vi "Cascade front panel.vi"() -> ()   [LabVIEW 2016]
uses:
  SDI-12/Sonde Vertical Graph.ctl
  Waterloo DAQ/controls/Vertical Chart.ctl
  activeXtest/activeXtest 2015 Folder/sample data row cluster.ctl
  activeXtest/activeXtest 2015 Folder/sonde cluster.ctl
  Groundwater header.ctl
  Waterloo DAQ/controls/MCC DAQ Setup.ctl
  Waterloo DAQ/controls/Aux Sensor.ctl
  KPRO_2016 subvis/Control 2.ctl
  KPRO_2016 subvis/Control 9.ctl
  KPRO_2016 subvis/Graph Controls 2.ctl
  KPRO_2016 subvis/Ik control.ctl
  KPRO_2016 subvis/Ion Slope Control 8.ctl
  KPRO_2016 subvis/Depth Control.ctl
  KPRO_2016 subvis/SS Control 7.ctl
  Waterloo DAQ/controls/Action Control 1.ctl
  <extravilib>/ChannelInstances/One Element Stream-t'Action Control 1.ctl'/Instantiate.vi
  <extravilib>/ChannelInstances/One Element Stream-t'Action Control 1.ctl'/Endpoint.vi
  <vilib>/ULx/Create Channel.llb/ULx Create Channel (AI-Voltage-Basic).vi
  <vilib>/ULx/Read.llb/ULx Read (Analog DBL 1Chan 1Samp).vi
  C:/Program Files (x86)/National Instruments/LabVIEW 2016/vi.lib/ULx/ULx_LV.dll
  <vilib>/Utility/NIReport.llb/NI_report.lvclass
  <vilib>/Utility/config.llb/NI_LVConfig.lvlib
  <extravilib>/ChannelInstances/One Element Stream-t'Action Control 1.ctl'.lvlib
panel:
  out "Feet of Stainless 2":i32
  out "Feet of\nStainless to be\nUsed (Count)":i32
  in  "SS In":i32
  in  "Record Continuous Samples":bool
  out "Current Time (s)":dbl
  in  "Sample Sheet Data Row Cluster 2":T1={"Head"=0.0, "Depth"=0.0, "comment string"="", "Sonde Data Cluster"={"Cumulative\nVolume"=100.0, "Specific\nConductance"=2.0, "Dissolved\nOxygen"=3.0, "pH"=4.0, "ORP"=5.0, "Temp"=26.0, "Salinity"=7.0}} {"Sonde Data Cluster"."Salinity" format="%_3g"; "Sonde Data Cluster"."Temp" format="%_2g"; "Sonde Data Cluster"."ORP" format="%_4g"; "Sonde Data Cluster"."pH" format="%_4g"; "Sonde Data Cluster"."Dissolved\nOxygen" format="%_4g"; "Sonde Data Cluster"."Specific\nConductance" format="%_4g"; "Sonde Data Cluster"."Cumulative\nVolume" format="%#_4g"}
  in  "stop":bool
  in  "Write Data to Spreadsheet":bool
  in  "Sample Not Collected":bool
  in  "Record Single Sample":bool
  in  "Tab Control":T3(tab)
  out "12V Voltage Monitor":dbl format="%_3f"
  out "Found Quanta Sonde Com Port":refnum<visa-resource-name>
  in  "Temporary Data Files Directory":path=path "D:/Cascade/Data/Raw Sonde Data"
  in  "Data File Directory":path=path "D:/Cascade/Data/Excel Reports"
  out "Quanta Sonde found?":bool
  in  "report file path":path=path "D:/Cascade/templates/Groundwater Profiling Log_empty_2.xlsx"
  in  "template file path":path=path "D:/Cascade/templates/Groundwater Profiling Log_empty_labview_template.xlsx"
  in  "Config File Path":path=path "D:/Cascade/Data/config files/DAQ Setup Config.ini"
  in  "Read Configuration File?":bool=TRUE
  out "H-4191 Adapter found":bool
  in  "Save Configuration File?":bool
  out "Sonde Communication Error Out":errorcluster
  in  "Search for Comm Ports?":bool=TRUE
  in  "USB Serial Port Manual Entry":refnum<visa-resource-name>="COM13"
  in  "MCC USB-DAQ Setup":T4={"Device Name in InstaCal"="Dev0", "Omega Pressure Sensor"={"DAQ Channel"=2.0, "Output Voltage Range"=1, "Enabled"=TRUE, "Description"="Uphole Pressure"}, "McMillian 102 Flowmeter"={"DAQ Channel"=11.0, "Output Voltage Range"=1, "Enabled"=TRUE, "Description"="Flow"}, "DHT Pressure Sensor"={"DAQ Channel"=3.0, "Output Voltage Range"=1, "Enabled"=TRUE, "Description"="Downhole Pressure"}, "Top String Pot"={"DAQ Channel"=0.0, "Output Voltage Range"=0, "Enabled"=TRUE, "Description"="Top String Pot"}, "String Pot Signal"={"DAQ Channel"=1.0, "Output Voltage Range"=0, "Enabled"=TRUE, "Description"="String Pot"}, "Aux Sensor 1"={"DAQ Channel"=5.0, "Output Voltage Range"=1, "Enabled"=FALSE, "Description"="Aux 1"}, "Aux Sensor 2"={"DAQ Channel"=6.0, "Output Voltage Range"=1, "Enabled"=FALSE, "Description"="Aux 2"}, "Aux Sensor 3"={"DAQ Channel"=7.0, "Output Voltage Range"=1, "Enabled"=TRUE, "Description"="Aux 3"}, "Voltage Monitor"={"DAQ Channel"=8.0, "Output Voltage Range"=0, "Enabled"=TRUE, "Description"="9V Monitor"}} {"Voltage Monitor"."Output Voltage Range" items=["+/-10 V Range", "+/-5 V Range", "+/-2.5V Range", "+/-1.25 V Range", "+/-0.625 V Range", "+/-0.3125 V Range", "+/-0.1562V Range", "+/-0.078125 V Range"]; "Aux Sensor 3"."Output Voltage Range" items=["+/-10 V Range", "+/-5 V Range", "+/-2.5V Range", "+/-1.25 V Range", "+/-0.625 V Range", "+/-0.3125 V Range", "+/-0.1562V Range", "+/-0.078125 V Range"]; "Aux Sensor 2"."Output Voltage Range" items=["+/-10 V Range", "+/-5 V Range", "+/-2.5V Range", "+/-1.25 V Range", "+/-0.625 V Range", "+/-0.3125 V Range", "+/-0.1562V Range", "+/-0.078125 V Range"]; "Aux Sensor 1"."Output Voltage Range" items=["+/-10 V Range", "+/-5 V Range", "+/-2.5V Range", "+/-1.25 V Range", "+/-0.625 V Range", "+/-0.3125 V Range", "+/-0.1562V Range", "+/-0.078125 V Range"]; "String Pot Signal"."Output Voltage Range" items=["+/-10 V Range", "+/-5 V Range", "+/-2.5V Range", "+/-1.25 V Range", "+/-0.625 V Range", "+/-0.3125 V Range", "+/-0.1562V Range", "+/-0.078125 V Range"]; "Top String Pot"."Output Voltage Range" items=["+/-10 V Range", "+/-5 V Range", "+/-2.5V Range", "+/-1.25 V Range", "+/-0.625 V Range", "+/-0.3125 V Range", "+/-0.1562V Range", "+/-0.078125 V Range"]; "DHT Pressure Sensor"."Output Voltage Range" items=["+/-10 V Range", "+/-5 V Range", "+/-2.5V Range", "+/-1.25 V Range", "+/-0.625 V Range", "+/-0.3125 V Range", "+/-0.1562V Range", "+/-0.078125 V Range"]; "McMillian 102 Flowmeter"."Output Voltage Range" items=["+/-10 V Range", "+/-5 V Range", "+/-2.5V Range", "+/-1.25 V Range", "+/-0.625 V Range", "+/-0.3125 V Range", "+/-0.1562V Range", "+/-0.078125 V Range"]; "Omega Pressure Sensor"."Output Voltage Range" items=["+/-10 V Range", "+/-5 V Range", "+/-2.5V Range", "+/-1.25 V Range", "+/-0.625 V Range", "+/-0.3125 V Range", "+/-0.1562V Range", "+/-0.078125 V Range"]}
  out "Rate":dbl=1000.0 caption="Sample Rate (Hz)"
  out "Number of Channels":u16
  in  "Channel Data Rate S/s":dbl=3720.0 format="%#_13g"
  out "Descriptions":string[](array[string])
  out "Raw Voltages":dbl[](array[numeric])
  out "9V Voltage Monitor":dbl
  in  "Record DAQ Raw Voltages":bool
  in  "Groundwater Header":T6
  out "Worksheet Names":string[](array[string])
  in  "Current Sheet":i32=1
  out "row max value":i32
  out "last occupied cell's name":string
  out "Current Sample Sheet":string="Sample 1"
  in  "Cluster":T7={"Profile ID"="WP-01", "Hole Id"="HOLE_001"}
  out "Sonde Data Array":string[][](array[string])
  out "Table Label":string="Data from Sample Sheet %d from Excel File"
  out "Sonde Data Display":T8
  out "Temperature":cluster{"Y":dbl[], "Y":dbl[]}[](graph)
  in  "Record Reason":bool
  in  "Select Reasons to Record Data":u16(ring) items=["Per Client Request", "Timed Out", "Sample stopped flowing", "Equipment Issue"]
  out "SC  Reference\nCalibrate Response":bool
  out "DO  Reference\nCalibrate Response":bool
  in  "Salinity \nReference":dbl
  out "Salinity  Reference\nCalibrate Response":bool
  out "ORP  Reference\nCalibrate Response":bool
  in  "SC \nReference":dbl
  in  "DO \nReference":dbl
  in  "ORP Reference":dbl
  in  "pH Reference":dbl
  in  "pH Zero":dbl
  in  "Record  SC Calibration":bool
  in  "Record DO Calibration":bool
  in  "Record Salinity Calibration":bool
  in  "Record ORP Calibration":bool
  in  "Record pH Calibration Reference":bool
  in  "Record pH Calibration Zero":bool
  out "pH Zero \nCalibrate Response":bool
  out "pH  Reference\nCalibrate Response":bool
  in  "Ion Offset":dbl format="%.2f"
  in  "Ion Slope":dbl=44.04 format="%.2f"
  in  "Pressure \nSlope":dbl=24.27199935913086 format="%.2f"
  in  "Flow Slope":dbl=37.99800109863281 format="%.2f"
  in  "String Pot \nSlope":dbl=1.7339999675750732 format="%.2f"
  out "Slug Test\nIndicator copy":bool
  out "KPRO Test\nIndicator":bool
  in  "Start\nST":bool
  in  "Finish Tests":bool
  in  "Start  KPRO":bool
  in  "Feet of Stainless":i32=40
  out "Cluster 7":T10={"Flow"=0.21081600494384767, "Zeroed \nPressure"=74.74207969932556, "Ik"=0.003788962123473114, "Current Depth"=-100.6, "Feet of Stainless"=40, "Start Depth"=0.0, "Hole_Name_Path"=path "C:/e"} {"Start Depth" format="%.2f"; "Current Depth" format="%.2f"; "Ik" format="%.2f"; "Zeroed \nPressure" format="%.2f"; "Flow" format="%.2f"}
  in  "Cluster 2":T11={"Ion Slope"=44.04, "Ion Offset"=0.0, "Height of Sample Box"=0.0, "Last_Pressure_Slope"=48.27000045776367, "Last_Flow_Slope"=39.040000915527344, "Last_String_Pot_Slope"=1.6619999408721924} {"Last_String_Pot_Slope" format="%.2f"; "Last_Flow_Slope" format="%.2f"; "Last_Pressure_Slope" format="%.2f"; "Height of Sample Box" format="%.2f"; "Ion Offset" format="%.2f"; "Ion Slope" format="%.2f"}
  in  "Slope Cluster":T12={"Total Volume"=0.0, "String Pot Slope"=1.6619999408721924, "Flow Slope"=39.040000915527344, "Pressure Slope"=48.27000045776367, "Depth to Water Table"=-0.0, "Atmospheric Pressure"=32.22022530555725, "Reservoir Pressure"=-0.004827000045779073} {"Reservoir Pressure" format="%.2f"; "Atmospheric Pressure" format="%.2f"; "Depth to Water Table" format="%.2f"; "Pressure Slope" format="%.2f"; "Flow Slope" format="%.2f"; "String Pot Slope" format="%.2f"; "Total Volume" format="%.2f"}
  in  "Cluster 6":T13
  out "Cluster 4":T14={"Real Time - Depth vs. lk "={[0.003788962123473114, 0.0037174584307500765, 0.0037174584307500765, 0.0037174584307500765, 0.0037174584307500765, 0.003788962123473114], [-100.1, -100.2, -100.3, -100.4, -100.5, -100.6]}, "Real Time - Depth vs. lk  2"={[0.003788962123473114, 0.0037174584307500765, 0.0037174584307500765, 0.0037174584307500765, 0.0037174584307500765, 0.003788962123473114], [-100.1, -100.2, -100.3, -100.4, -100.5, -100.6]}, "Real Time - Depth vs. lk  2"={[0.003788962123473114, 0.0037174584307500765, 0.0037174584307500765, 0.0037174584307500765, 0.0037174584307500765, 0.003788962123473114], [-100.1, -100.2, -100.3, -100.4, -100.5, -100.6]}, "Ik "=0.003788962123473114, "Current Depth"=-100.6} {"Current Depth" format="%.2f"; "Ik" format="%.2f"}
  in  "Cluster 3":T15={"Cumulative - Depth vs. Ik"={[], []}, "Real Time - Depth vs. lk "={[0.003788962123473114, 0.0037174584307500765, 0.0037174584307500765, 0.0037174584307500765, 0.0037174584307500765, 0.003788962123473114], [-100.1, -100.2, -100.3, -100.4, -100.5, -100.6]}, "Cumulative - Depth vs. Drive"={[], []}, "Real Time - Depth vs. Drive"={[0.02036245163917736, 0.125, 0.16666666666666674, 0.16666666666666663, 0.16666666666666663, 0.16666666666666663], [-100.1, -100.2, -100.3, -100.4, -100.5, -100.6]}}
  out "DAQ Error":errorcluster
  out "Initialization Finished":bool=TRUE
  out "Stop":bool
  out "error out":errorcluster
  in  "error in (no error)":errorcluster
  out "producer loop":i32
  out "consumer loop":i32
  out "Active Channel Array":string[](array[string])
  out "delimited string":string
  out "Voltage Range":dbl[](array[numeric])
  out "Stop 2":bool
  # "Instructions for Sonde Calibration:\n1.  Use the Record Single Point to Record the Data prior to start of\ncalibration procedure to record the initial points to the excel worksheet.\n2.  pH Calibration is a 2 step process:  A pH standard between 6.8 and 7.2 is treated as the “zero”\nand all other values are treated as the “slope”. First calibrate “zero”, then  add a second to calibrate “slope”. \n3.  Specific Conductance:  Wait for the specific conductance readings to stabilize in the calibration solution, which may\nrequire one or two minutes."
  # "String Pot"
  # "Use Incr"
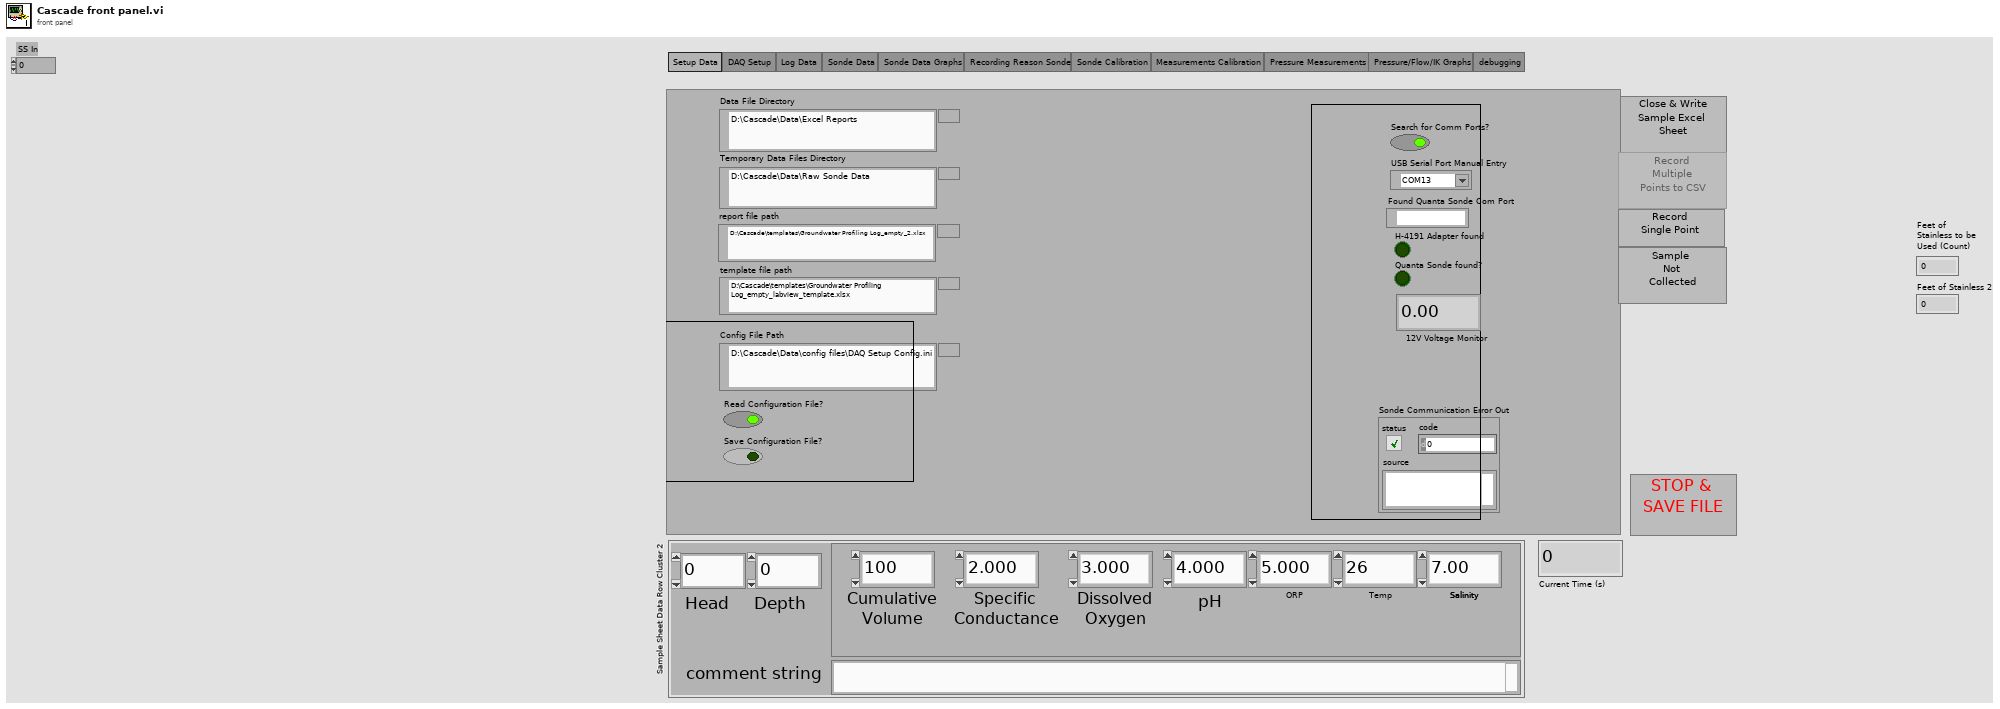
[diagram p1: front panel]
types:
  T1 = typedef "sample data row cluster.ctl" = cluster{"Head":dbl, "Depth":dbl, "comment string":string, "Sonde Data Cluster":T2}
  T2 = typedef "sonde cluster.ctl" = cluster{"Cumulative\nVolume":dbl, "Specific\nConductance":dbl, "Dissolved\nOxygen":dbl, "pH":dbl, "ORP":dbl, "Temp":dbl, "Salinity":dbl}
  T3 = enum32{"Setup Data", "DAQ Setup", "Log Data", "Sonde Data", "Sonde Data Graphs", "Recording Reason Sonde", "Sonde Calibration", "Measurements Calibration", "Pressure Measurements", "Pressure/Flow/IK Graphs", "debugging"}
  T4 = typedef "MCC DAQ Setup.ctl" = cluster{"Device Name in InstaCal":string, "Omega Pressure Sensor":T5, "McMillian 102 Flowmeter":T5, "DHT Pressure Sensor":T5, "Top String Pot":T5, "String Pot Signal":T5, "Aux Sensor 1":T5, "Aux Sensor 2":T5, "Aux Sensor 3":T5, "Voltage Monitor":T5}
  T5 = typedef "Aux Sensor.ctl" = cluster{"DAQ Channel":dbl, "Output Voltage Range":u16, "Enabled":bool, "Description":string}
  T6 = typedef "Groundwater header.ctl" = cluster{"Location":string, "Date Finished":string, "CTS":string, "sampler":string, "Kpro box Serial ":string, "Sonde Serial":string, "Drilling Contractor":string, "Ave Depth to Water":string, "Gas/Peri Pump":string, "Atmospheric Pressure":string, "KPRO N2 Pressure":string, "Gas Drive N2 Pressure":string}
  T7 = typedef "Control 9.ctl" = cluster{"Profile ID":string, "Hole Id":string}
  T8 = typedef "Sonde Vertical Graph.ctl" = cluster{"pH":T9, "Conductance":T9, "Salinity":T9, "DO % Saturation":T9, "DO mg/L":T9, "ORP":T9}
  T9 = typedef "Vertical Chart.ctl" = cluster{"Y":dbl[], "Y":dbl[]}[]
  T10 = typedef "SS Control 7.ctl" = cluster{"Flow":dbl, "Zeroed \nPressure":dbl, "Ik":dbl, "Current Depth":sgl, "Feet of Stainless":i32, "Start Depth":sgl, "Hole_Name_Path":path}
  T11 = typedef "Ion Slope Control 8.ctl" = cluster{"Ion Slope":dbl, "Ion Offset":dbl, "Height of Sample Box":dbl, "Last_Pressure_Slope":dbl, "Last_Flow_Slope":dbl, "Last_String_Pot_Slope":dbl}
  T12 = typedef "Control 2.ctl" = cluster{"Total Volume":dbl, "String Pot Slope":dbl, "Flow Slope":dbl, "Pressure Slope":dbl, "Depth to Water Table":dbl, "Atmospheric Pressure":dbl, "Reservoir Pressure":dbl}
  T13 = typedef "Depth Control.ctl" = cluster{"Depth mode":bool, "Increment\nButton":bool}
  T14 = typedef "Ik control.ctl" = cluster{"Real Time - Depth vs. lk ":cluster{dbl[], dbl[]}, "Real Time - Depth vs. lk  2":cluster{dbl[], dbl[]}, "Real Time - Depth vs. lk  2":cluster{dbl[], dbl[]}, "Ik ":dbl, "Current Depth":sgl}
  T15 = typedef "Graph Controls 2.ctl" = cluster{"Cumulative - Depth vs. Ik":cluster{dbl[], dbl[]}, "Real Time - Depth vs. lk ":cluster{dbl[], dbl[]}, "Cumulative - Depth vs. Drive":cluster{dbl[], dbl[]}, "Real Time - Depth vs. Drive":cluster{dbl[], dbl[]}}
  T16 = typedef "Action Control 1.ctl" = enum16{"TimeOut", "Continuous  Data", "Init", "Exit", "Acq. Single Point", "Write Sample Sheet", "Acq. DAQ data", "Sample Not Collected", "Record Reason", "pH Calibration Zero", "pH Calibration Standard", "ORP Calibration Standard", "Salinity Calibration Standard", "DO Calibration Standard", "SC Calibration Standard"}
  T17 = typedef "NI_LVConfig.lvlib/Config Data RefNum.ctl" = refnum<k1>
  T18 = enum8{"Enabled", "Disabled", "Disabled and Grayed Out"}
  T19 = typedef "One Element Stream-t'Action Control 1.ctl'.lvlib/)Channel.ctl" = refnum<queue>
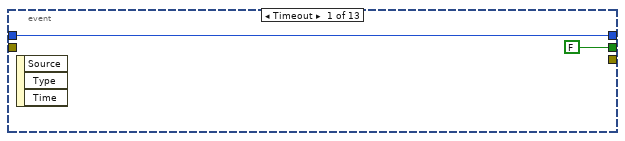
[diagram p2: hidden frame]
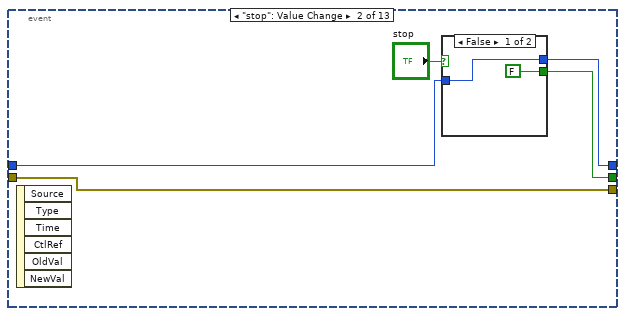
[diagram p3: hidden frame]
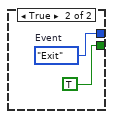
[diagram p4: hidden frame]
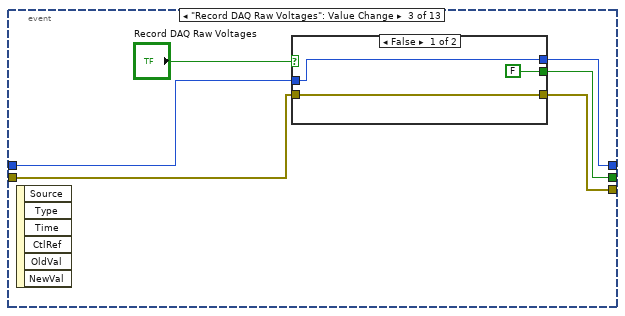
[diagram p5: hidden frame]
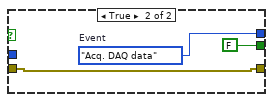
[diagram p6: hidden frame]
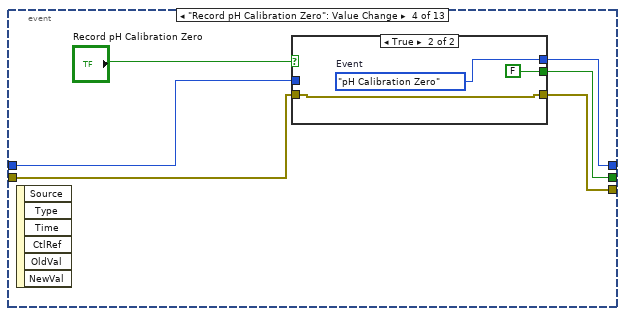
[diagram p7: hidden frame]
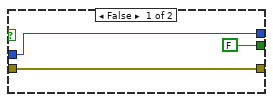
[diagram p8: hidden frame]
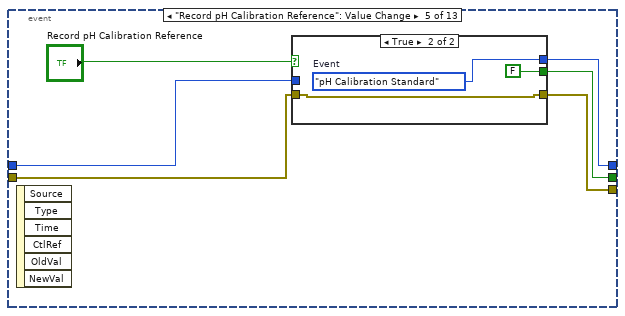
[diagram p9: hidden frame]
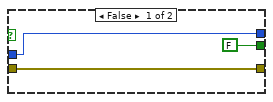
[diagram p10: hidden frame]
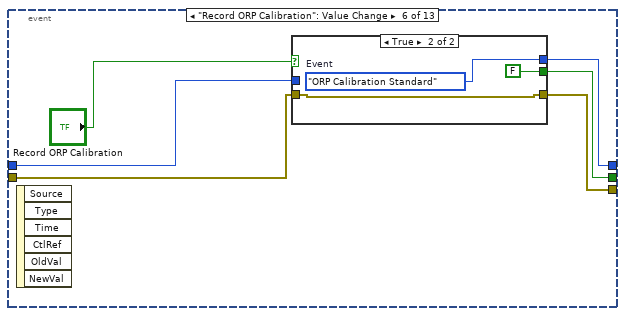
[diagram p11: hidden frame]
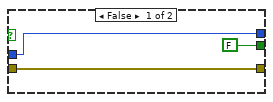
[diagram p12: hidden frame]
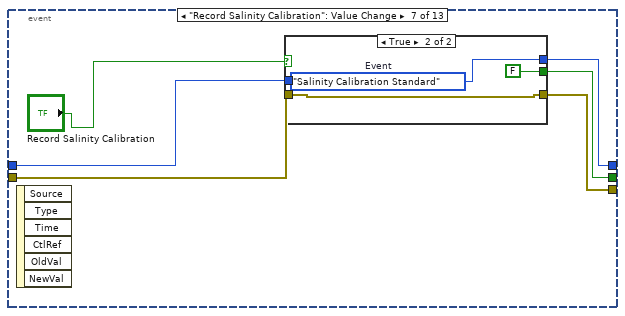
[diagram p13: hidden frame]
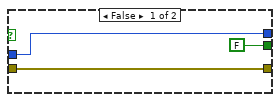
[diagram p14: hidden frame]
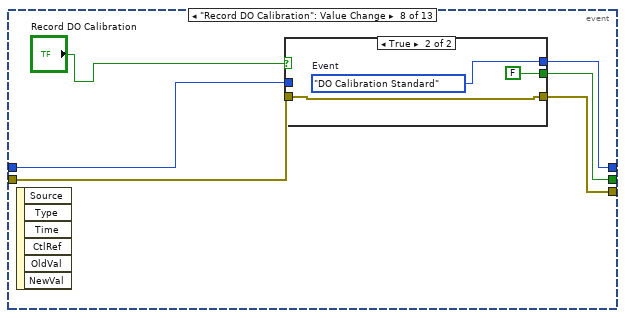
[diagram p15: hidden frame]
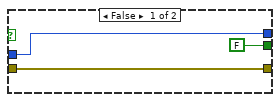
[diagram p16: hidden frame]
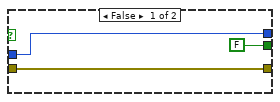
[diagram p17: hidden frame]
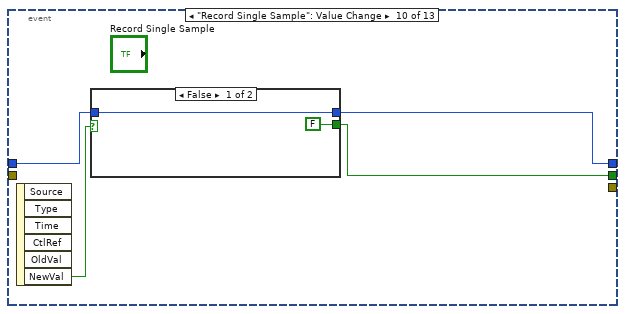
[diagram p18: hidden frame]
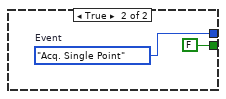
[diagram p19: hidden frame]
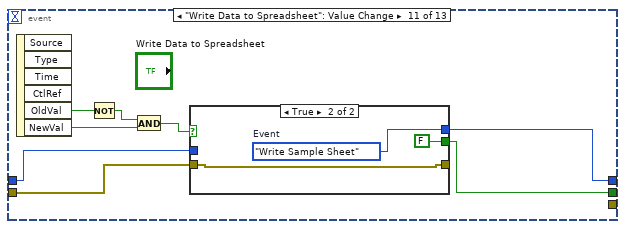
[diagram p20: hidden frame]
diagram:
  w7 = Action_Control_1."Init"  # Event
  # "For calibrate command (XC) on SDI-12 address ‘a’, P is pH, C is specific conductance, S is\nsalinity or TDS, % is DO %Saturation, O is DO mg/L, R is ORP, D is depth, B is\nbarometric pressure, and t is TDS scale factor."
  n1 = flat-sequence {
    tunnel: [w31] -> w10
    tunnel: [w63] -> w16
    tunnel: w10 -> [w63]
    tunnel: [w59] -> w6
    tunnel: [w74] -> w26
    tunnel: w16 -> [w71]
    tunnel: [w71] -> w11
    tunnel: w26 -> [w130]
    tunnel: [w102] -> w24
    tunnel: [w106] -> w22
    tunnel: [w113] -> w17
    tunnel: [w112] -> w19
    tunnel: [w111] -> w20
    tunnel: [w104] -> _
    tunnel: [w100] -> w25
    tunnel: ["Feet of Stainless"] -> w5
    tunnel: [w97] -> w4
    tunnel: [w96] -> w3
    frame #0 {
      n2 = flat-sequence {
        tunnel: [w35] -> w31
        tunnel: "error in (no error)" -> [w34]
        frame #0 {
          n3 = case shown="False" "Read Configuration File?" {
            selector: "Read Configuration File?" -> [_ w42]
            tunnel: [w36 w47] -> w35
            tunnel: w34 -> [w36 w44]
            tunnel: "Config File Path" -> [_ w43]
            frame False {
            }
            frame True {
              n4 = call <vilib>:"Check if File or Folder Exists.vi"("error in (no error)"=w44, "path"=w43) -> ("error out"=w39:errorcluster, "file or folder exists?"=w40:bool, "dup path"=w38:path)  [unwired: 7 in]
              n5 = And(x=w42, y=w40) -> (x .and. y?=w41:bool)
              n6 = control-ref of="This VI"() -> (w45:refnum<vi>)
              n7 = case shown="True" w41 {
                selector: w41 -> [w48 _]
                tunnel: w38 -> [_ w53]
                tunnel: w39 -> [w49 w57]
                tunnel: [w49 w50] -> w46
                tunnel: w45 -> [_ w58]
                frame False {
                  n8 = local write "Read Configuration File?"(w48) -> ()
                }
                frame True {
                  n9 = call <vilib>:"Open Config Data.vi"("error in (no error)"=w57, "create file if necessary (T)"=FALSE, "configuration file path"=w53) -> ("error out"=w55:errorcluster, "refnum"=w56:T17)  [unwired: 6 in, 1 out]
                  n10 = call <userlib>:"Read Panel from INI__ogtk.vi"("error in (no error)"=w55, "VI ref"=w58, "refnum"=w56) -> ("error out"=w51:errorcluster, "refnum out"=w52:T17)  [unwired: 7 in]
                  n11 = call <vilib>:"Close Config Data.vi"("error in (no error)"=w51, "refnum"=w52) -> ("error out"=w50:errorcluster)  [unwired: 8 in, 1 out]
                }
              }
              n12 = call <vilib>:"Clear Errors.vi"("error in (no error)"=w46) -> ("error out"=w37:errorcluster)  [unwired: 5 in, 1 out]
              n13 = Merge Errors(w37) -> (w47:errorcluster)
            }
          }
        }
      }
      n14 = invoke on="error out" class="Clust (strict)" method="Reinit To Default"(error in="error in (no error)") -> ()  [unwired: 2 in, 3 out]
    }
    frame #1 {
      n15 = Get Date/Time In Seconds() -> (seconds since 1Jan1904=w60:timestamp)
      n16 = Get Date/Time In Seconds() -> (seconds since 1Jan1904=w59:timestamp)
      n17 = local write "Current Sheet"(1 ("Current Sheet")) -> ()
      n18 = Subtract(x=w59, y=w60) -> (x-y=w61:dbl)
      n19 = To Double Precision Float(number=w61) -> (double precision float=→"Current Time (s)":dbl)
    }
    frame #2 {
      w83 = T18."Disabled and Grayed Out" ("Disabled")
      (unwired) FALSE ("Stop")
      n20 = control-ref of="Sonde Data Display"() -> ()  [unwired: 1 out]
      n21 = invoke on="Current Sheet" class="DigNum (strict)" method="Reinit To Default"() -> (error out=w76:errorcluster)  [unwired: 3 in, 2 out]
      n22 = local write "Initialization Finished"(FALSE ("Initialization Finished")) -> ()
      n23 = local write "Groundwater Header"(T6 {"Location"="Randolph VT", "Date Finished"="", "CTS"="123456789", "sampler"="MM", "Kpro box Serial "="12345", "Sonde Serial"="Quanta ", "Drilling Contractor"="ARA", "Ave Depth to Water"="0.00", "Gas/Peri Pump"="Peri", "Atmospheric Pressure"="760mm", "KPRO N2 Pressure"="69.35psi", "Gas Drive N2 Pressure"="NA"} ("Groundwater Header 2")) -> ()
      n24 = invoke on="Sample Not Collected" class="Bool" method="Reinit To Default"(error in=w76) -> (error out=w80:errorcluster)  [unwired: 2 in, 2 out]
      n25 = invoke on="Record Continuous Samples" class="Bool" method="Reinit To Default"(error in=w80) -> (error out=w79:errorcluster)  [unwired: 2 in, 2 out]
      n26 = property on="Record Continuous Samples" class="Bool"("DisabledEnum"=w83) -> (error out=w84:errorcluster)  [unwired: 2 in, 1 out]
      n27 = call "search for Quanta Sonde devices.vi"("VISA resource name"="USB Serial Port Manual Entry", "Search for Comm Ports?"="Search for Comm Ports?", "error in (no error)"=w71) -> ("12V monitor"=→"12V Voltage Monitor":dbl, "Com Port with Quanta Sonde devices"=w90:refnum<visa-resource-name>[], "Number of Quanta Sonde devices"=w89:i32, "Number of Quanta Sonde devices > 0?"=→"Quanta Sonde found?":bool, "H-4191 Adapter found"=→"H-4191 Adapter found":bool, "Error Out"=w68:errorcluster)  [unwired: 5 in, 2 out]
      "Sonde Communication Error Out" <- w68
      n28 = case shown="0, Default" w89 {
        tunnel: w90 -> [_ w95]
        tunnel: [refnum<visa-resource-name> refnum ("RS232 Port Out") w93] -> w88
        frame 0, Default {
        }
        frame 1 {
          n29 = Index Array(array=w95, index=0) -> (element=w93:refnum<visa-resource-name>)
        }
      }
      "Found Quanta Sonde Com Port" <- w88
      n30 = invoke on="Write Data to Spreadsheet" class="Bool" method="Reinit To Default"(error in=w79) -> (error out=w78:errorcluster)  [unwired: 2 in, 2 out]
      n31 = property on="Record Single Sample" class="Bool"(error in=w84, "DisabledEnum"=w83) -> (error out=w85:errorcluster)  [unwired: 1 in, 1 out]
      n32 = invoke on="Record Single Sample" class="Bool" method="Reinit To Default"(error in=w78) -> (error out=w77:errorcluster)  [unwired: 2 in, 2 out]
      n33 = call <vilib>:"Clear Errors.vi"("error in (no error)"=w68) -> ("error out"=w67:errorcluster)  [unwired: 5 in, 1 out]
      n34 = invoke on="stop" class="Bool" method="Reinit To Default"(error in=w77) -> (error out=w82:errorcluster)  [unwired: 2 in, 2 out]
      n35 = invoke on="Stop" class="Bool (strict)" method="Reinit To Default"() -> (error out=w70:errorcluster)  [unwired: 3 in, 2 out]
      n36 = property on="Write Data to Spreadsheet" class="Bool"(error in=w82, "DisabledEnum"=w83) -> (error out=w73:errorcluster)  [unwired: 1 in, 1 out]
      n37 = property on="Sample Not Collected" class="Bool"(error in=w85, "DisabledEnum"=w83) -> (error out=w81:errorcluster)  [unwired: 1 in, 1 out]
      n38 = invoke on="Stop 2" class="Bool (strict)" method="Reinit To Default"(error in=w70) -> (error out=w69:errorcluster)  [unwired: 2 in, 2 out]
      n39 = Merge Errors(w67, w69, w73, w81) -> (w74:errorcluster)
    }
    frame #3 {
      w105 = "Sample 1" ("Worksheet Name in")
      n40 = flat-sequence {
        frame #0 {
        }
      }
      n41 = call "get sample header columns.vi"("error in (no error)"=w130) -> ("Column of Volume"=w112:i32, "Columns"=w111:i32[], "data"=w123:string[][], "error out"=w131:errorcluster)  [unwired: 5 in, 6 out]
      n42 = call "close excel file if open.vi"("error in (no error)"=w131, "report file path in"="report file path") -> ("error out"=w116:errorcluster, "report file path out"=w99:path)  [unwired: 8 in]
      n43 = Index Array(array=w123, index (col)=0 ("disabled index (col)")) -> (element=w122:string[])  [unwired: 1 in]
      n44 = flat-sequence {
        tunnel: [w132] -> w96
        frame #0 {
          n45 = Unbundle By Name("Slope Cluster") -> ("Depth to Water Table"=w135:dbl)
          n46 = call "New Stainless Correction Pop Up 2016.vi"("New Feet\n of Stainless\n(Count)"="SS In", "Depth to \nWater Table\nInput"=w135) -> ("Feet of\nStainless to be\nUsed (Count)"=w132:i32, "Depth to \nWater Table\nOutput"=w133:dbl)  [unwired: 2 in]
          n47 = Bundle By Name(cluster="Slope Cluster", "Depth to Water Table"=w133) -> (w136:T12)
          n48 = local write "Slope Cluster"(w136) -> ()
        }
      }
      n49 = call "copy excel template.vi"("error in (no error)"=w116, "report file path in"=w99, "template file path in"="template file path") -> ("error out"=w117:errorcluster, "report file path out"=w119:path)  [unwired: 7 in]
      n50 = Array Size(array=w122) -> (size(s)=w129:i32)
      n51 = Initialize Array("", 10 ("dimension size"), w129) -> (w127:string[][])
      n52 = call "open excel get worksheet names.vi"("error in (no error)"=w117, "milliseconds to wait"=u32 5, "report file path"=w119) -> ("error out"=w114:errorcluster, "Number of Sample Sheets"=w113:i32, "NI_report out"=w115:refnum<class "NI_report.lvclass">, "Worksheet Names"=w106:string[])  [unwired: 3 in, 2 out]
      "Worksheet Names" <- w106
      n53 = flat-sequence {
        tunnel: w114 -> [w160]
        tunnel: [w159] -> w108
        tunnel: [w156] -> w109
        tunnel: [w158] -> _
        tunnel: w106 -> [w157]
        tunnel: w115 -> [w156]
        frame #0 {
          n54 = call "groundwater log header.vi"("Worksheet Names"=w157, "Groundwater Header"="Groundwater Header", "error in (no error)"=w160, "NI_report in"=w156) -> ("error out"=w159:errorcluster, "NI_report out"=w158:refnum<class "NI_report.lvclass">)  [unwired: 6 in]
        }
      }
      n55 = Insert Into Array(array=w127, index (row)=0, new element=w122) -> (→"Sonde Data Array":string[][])  [unwired: 1 in]
      n56 = flat-sequence {
        tunnel: [w138] -> w97
        frame #0 {
          # "KPRO Array"
          n57 = Initialize Array(0.0, 0, 9) -> (w138:dbl[][])
        }
      }
      n58 = local write "Current Sample Sheet"(w105) -> ()
      n59 = call "find and open select worksheet.vi"("Worksheet Names"=w106, "error in (no error)"=w108, "milliseconds to wait"=u32 100, "Worksheet Name in"=w105, "NI_report in"=w109) -> ("error out"=w101:errorcluster, "Select Worksheet Index"=w104:i32, "NI_report out"=w103:refnum<class "NI_report.lvclass">)  [unwired: 4 in]
      n60 = flat-sequence {
        tunnel: w101 -> [w155]
        tunnel: w103 -> [w154]
        tunnel: [w153] -> w102
        tunnel: [w147] -> w100
        tunnel: [w145] -> _
        frame #0 {
          (unwired) 3 ("Header Rows to remove")
          n61 = local read "Current Sample Sheet"() -> (w143:string)
          n62 = call "get sample sheet data cells.vi"("error in (no error)"=w155, "NI_report in"=w154) -> ("error out"=w148:errorcluster, "data"=w149:string[][], "NI_report out"=w153:refnum<class "NI_report.lvclass">, "left edge output cluster"=w146:cluster{"row":i32, "column":i32})  [unwired: 5 in, 1 out]
          n63 = call "find last occupied cell.vi"("data"=w149, "Active Sheet"=w143, "Header Rows to remove"=3, "sub array start"=w146, "error in (no error)"=w148) -> ("row max value"=w144:i32, 13:"start of last occupied row"=w145:cluster{"row":i32, "column":i32}, 14:"start of last occupied row"=w142:string, "error out"=w147:errorcluster)  [unwired: 4 in, 3 out]
          n64 = Array Subset(array=w149, index (col)=2 ("index")) -> (w151:string[][])  [unwired: 3 in]
          n65 = local write "Sonde Data Array"(w151) -> ()
          n66 = local write "row max value"(w144) -> ()
          n67 = local write "last occupied cell's name"(w142) -> ()
        }
      }
    }
  }
  n68 = while {
    shift-right: [w169] -> w29
    shift-left: w25 -> [w169]
    shift-right: [w164] -> _
    shift-left: w7 -> [w162]
    tunnel: [w170] -> w9
    i -> [w168]
    stop <- w166 stop-if-true
    # "User Interface Producer Loop"
    n69 = First Call?() -> (First Call?: T/F=w163:bool)
    n70 = case shown="False" w163 {
      tunnel: w169 -> [w175 _]
      tunnel: [w173 FALSE ("Boolean")] -> w166
      tunnel: [w172 w310] -> w164
      tunnel: w162 -> [_ w310]
      frame False {
        w171 = Action_Control_1."TimeOut"  # Event
        n71 = event shown="[8] \"Record  SC Calibration\": Value Change" {
          selector: _ -> [_ _ _ _ _ _ _ _ _ _ _ _ _]
          dyn-events: _ -> [_ _ _ _ _ _ _ _ _ _ _ _ _]
          timeout: 100 -> [_ _ _ _ _ _ _ _ _ _ _ _ _]
          tunnel: [w176 w182 w188 w201 w213 w225 w237 w249 w261 w274 w285 w295 w303] -> w172
          tunnel: [FALSE w181 w189 w202 w214 w226 w238 w250 w262 w273 w284 w296 w304] -> w173
          tunnel: w175 -> [_ w179 w191 w204 w216 w228 w240 w252 w264 _ w281 _ _]
          tunnel: [_ w179 w190 w203 w215 w227 w239 w251 w263 _ _ _ _] -> _
          tunnel: w171 -> [w176 w178 w187 w200 w212 w224 w236 w248 w260 w271 w279 w293 w301]
          event Timeout {
            n72 = event-data() -> ()  [unwired: 1 in, 3 out]
          }
          event "stop": Value Change {
            n73 = event-data() -> ()  [unwired: 1 in, 6 out]
            n74 = case shown="False" "stop" {
              tunnel: [w183 w185] -> w182
              tunnel: [FALSE TRUE] -> w181
              tunnel: w178 -> [w183 _]
              frame False {
              }
              frame True {
                w185 = Action_Control_1."Exit"  # Event
              }
            }
          }
          event "Record DAQ Raw Voltages": Value Change {
            n75 = event-data() -> ()  [unwired: 1 in, 6 out]
            n76 = case shown="False" "Record DAQ Raw Voltages" {
              tunnel: [w193 w196] -> w188
              tunnel: [FALSE FALSE ("Boolean")] -> w189
              tunnel: [w194 w197] -> w190
              tunnel: w191 -> [w194 w197]
              tunnel: w187 -> [w193 _]
              frame False {
              }
              frame True {
                w196 = Action_Control_1."Acq. DAQ data"  # Event
              }
            }
          }
          event "Record pH Calibration Zero": Value Change {
            n77 = event-data() -> ()  [unwired: 1 in, 6 out]
            n78 = case shown="True" "Record pH Calibration Zero" {
              tunnel: [w205 w208] -> w201
              tunnel: [FALSE FALSE ("Boolean")] -> w202
              tunnel: [w206 w209] -> w203
              tunnel: w204 -> [w206 w209]
              tunnel: w200 -> [w205 _]
              frame False {
              }
              frame True {
                w208 = Action_Control_1."pH Calibration Zero"  # Event
              }
            }
          }
          event "Record pH Calibration Reference": Value Change {
            n79 = event-data() -> ()  [unwired: 1 in, 6 out]
            n80 = case shown="True" "Record pH Calibration Reference" {
              tunnel: [w217 w220] -> w213
              tunnel: [FALSE FALSE ("Boolean")] -> w214
              tunnel: [w218 w221] -> w215
              tunnel: w216 -> [w218 w221]
              tunnel: w212 -> [w217 _]
              frame False {
              }
              frame True {
                w220 = Action_Control_1."pH Calibration Standard"  # Event
              }
            }
          }
          event "Record ORP Calibration": Value Change {
            n81 = event-data() -> ()  [unwired: 1 in, 6 out]
            n82 = case shown="True" "Record ORP Calibration" {
              tunnel: [w229 w232] -> w225
              tunnel: [FALSE FALSE ("Boolean")] -> w226
              tunnel: [w230 w233] -> w227
              tunnel: w228 -> [w230 w233]
              tunnel: w224 -> [w229 _]
              frame False {
              }
              frame True {
                w232 = Action_Control_1."ORP Calibration Standard"  # Event
              }
            }
          }
          event "Record Salinity Calibration": Value Change {
            n83 = event-data() -> ()  [unwired: 1 in, 6 out]
            n84 = case shown="True" "Record Salinity Calibration" {
              tunnel: [w241 w244] -> w237
              tunnel: [FALSE FALSE ("Boolean")] -> w238
              tunnel: [w242 w245] -> w239
              tunnel: w240 -> [w242 w245]
              tunnel: w236 -> [w241 _]
              frame False {
              }
              frame True {
                w244 = Action_Control_1."Salinity Calibration Standard"  # Event
              }
            }
          }
          event "Record DO Calibration": Value Change {
            n85 = event-data() -> ()  [unwired: 1 in, 6 out]
            n86 = case shown="True" "Record DO Calibration" {
              tunnel: [w253 w256] -> w249
              tunnel: [FALSE FALSE ("Boolean")] -> w250
              tunnel: [w254 w257] -> w251
              tunnel: w252 -> [w254 w257]
              tunnel: w248 -> [w253 _]
              frame False {
              }
              frame True {
                w256 = Action_Control_1."DO Calibration Standard"  # Event
              }
            }
          }
          event "Record  SC Calibration": Value Change {
            n87 = event-data() -> ()  [unwired: 1 in, 6 out]
            n88 = case shown="True" "Record  SC Calibration" {
              tunnel: [w265 w268] -> w261
              tunnel: [FALSE FALSE ("Boolean")] -> w262
              tunnel: [w266 w269] -> w263
              tunnel: w264 -> [w266 w269]
              tunnel: w260 -> [w265 _]
              frame False {
              }
              frame True {
                w268 = Action_Control_1."SC Calibration Standard"  # Event
              }
            }
          }
          event "Record Single Sample": Value Change {
            n89 = event-data() -> ("NewVal"=w272:bool)  [unwired: 1 in, 5 out]
            n90 = case shown="False" w272 {
              tunnel: [w275 w277] -> w274
              tunnel: [FALSE FALSE] -> w273
              tunnel: w271 -> [w275 _]
              frame False {
              }
              frame True {
                w277 = Action_Control_1."Acq. Single Point"  # Event
              }
            }
          }
          event "Write Data to Spreadsheet": Value Change {
            n91 = event-data() -> ("OldVal"=w283:bool, "NewVal"=w286:bool)  [unwired: 1 in, 4 out]
            n92 = Not(x=w283) -> (.not. x?=w282:bool)
            n93 = And(x=w282, y=w286) -> (x .and. y?=w280:bool)
            n94 = case shown="True" w280 {
              tunnel: [w287 w290] -> w285
              tunnel: [FALSE FALSE ("Boolean")] -> w284
              tunnel: [w288 w291] -> _
              tunnel: w281 -> [w288 w291]
              tunnel: w279 -> [w287 _]
              frame False {
              }
              frame True {
                w290 = Action_Control_1."Write Sample Sheet"  # Event
              }
            }
          }
          event "Sample Not Collected": Value Change {
            n95 = event-data() -> ("NewVal"=w294:bool)  [unwired: 1 in, 5 out]
            n96 = case shown="True" w294 {
              tunnel: [FALSE FALSE] -> w296
              tunnel: [w297 w299] -> w295
              tunnel: w293 -> [_ w299]
              frame True {
                w297 = Action_Control_1."Sample Not Collected"  # Event
              }
              frame False {
              }
            }
          }
          event "Record Reason": Value Change {
            n97 = event-data() -> ("NewVal"=w302:bool)  [unwired: 1 in, 5 out]
            n98 = case shown="True" w302 {
              tunnel: [FALSE FALSE] -> w304
              tunnel: [w305 w307] -> w303
              tunnel: w301 -> [_ w307]
              frame True {
                w305 = Action_Control_1."Record Reason"  # Event
              }
              frame False {
              }
            }
          }
        }
      }
      frame True {
      }
    }
    "Stop" <- w166
    n99 = local read "Stop"() -> (w167:bool)
    n100 = Or(x=w167, y=w166) -> ()  [unwired: 1 out]
    n101 = call <extravilib>:"Write With Abort.vi"("abort"=FALSE, "last element? (F)"=w166, "element"=w164) -> ("channel"=w170:T19)  [unwired: 6 in, 2 out]
    "producer loop" <- w168
  }
  n102 = Get Date/Time In Seconds() -> (seconds since 1Jan1904=w13:timestamp)
  n103 = To Double Precision Float(number=w13) -> (double precision float=w12:dbl)
  n104 = while {
    tunnel: w25 -> [w347]
    tunnel: [w349] -> w28
    tunnel: w9 -> [w319]
    tunnel: w24 -> [w346]
    shift-right: [w334] -> _
    shift-left: "Current Sheet" -> [w340]
    tunnel: w22 -> [w336]
    tunnel: w20 -> [w344]
    tunnel: w19 -> [w343]
    shift-right: [w335] -> _
    shift-left: 0 ("row index") -> [w342]
    tunnel: [w341] -> _
    shift-right: [w339] -> _
    shift-left: cluster{"row":i32, "column":i32} {"row"=0, "column"=0} ("start of last occupied row") -> [w338]
    tunnel: w17 -> [w333]
    shift-right: [w327] -> _
    shift-left: dbl[] [] ("Time Array") -> [w328]
    shift-right: [w326] -> _
    shift-left: dbl[][] [] ("Time Array") -> [w325]
    tunnel: w12 -> [w324]
    tunnel: [w322] -> _
    tunnel: w11 -> [w321]
    shift-right: [w317] -> _
    shift-left: refnum<k24>[] [] -> [w323]
    tunnel: w6 -> [w315]
    shift-right: [w314] -> w1
    shift-left: w5 -> [w314]
    tunnel: w4 -> [_]
    shift-right: [w313] -> w2
    shift-left: w3 -> [w313]
    i -> [w348]
    stop <- w320 stop-if-true
    # "Consumer Data Handling Loop"
    n105 = call <extravilib>:"Read With Abort.vi"("abort"=FALSE, "channel"=w319) -> ("last element?"=w318:bool, "element"=w330:T16)  [unwired: 5 in, 3 out]
    n106 = call <userlib>:"Wait (ms)__ogtk.vi"("error in (no error)"=w347, "milliseconds to wait"=u32 50) -> ("error out"=w332:errorcluster)  [unwired: 8 in, 1 out]
    n107 = feedback-in #1(w330) -> ()
    n108 = feedback #1() -> (w329:T16)  [unwired: 1 in]
    n109 = flat-sequence {
      frame #0 {
        n110 = call "Get_SLOPE_data_from_file 2016.vi"() -> ()  [unwired: 8 in, 4 out]
        n111 = call "Pressure 2016.vi"() -> ()  [unwired: 3 in, 1 out]
        n112 = call "In-Line-Pressure 2016.vi"() -> ()  [unwired: 11 in, 1 out]
        n113 = call "boolean debounce 2016.vi"() -> ()  [unwired: 1 in, 1 out]
        n114 = call "Flow 2016.vi"() -> ()  [unwired: 9 in, 1 out]
      }
    }
    n115 = call "open select sample sheet.vi"("Number of Sample Sheets"=w333, "error in (no error)"=w332, "Worksheet Names"=w336, "Active Sample Sheet"=w340, "NI_report in"=w346) -> ("error out"=w312:errorcluster, "Current Sample Sheet"=w316:string, "NI_report out"=w345:refnum<class "NI_report.lvclass">)  [unwired: 3 in, 1 out]
    n116 = flat-sequence {
      tunnel: w316 -> [w358]
      tunnel: w315 -> [w353]
      tunnel: w312 -> [w352]
      tunnel: [w350] -> w311
      frame #0 {
        n117 = Get Date/Time In Seconds() -> (seconds since 1Jan1904=w354:timestamp)
        n118 = Scan From String(format string="Sample %d", input string=w358, error in=w352) -> (error out=w351:errorcluster, output 1=w356:i32)  [unwired: 2 in, 2 out]
        n119 = Subtract(x=w354, y=w353) -> (x-y=w355:dbl)
        n120 = Format Into String(format string="Data from Sample Sheet %d from Excel File", error in=w351, w356) -> (resulting string=→"Table Label":string, error out=w350:errorcluster)  [unwired: 1 in]
        n121 = local write "Current Time (s)"(w355) -> ()
        "Current Sample Sheet" <- w358
      }
    }
    n122 = case shown="\"Salinity Calibration Standard\"" w330 {
      selector: w330 -> [_ _ _ _ _ _ _ _ _ _ _ w1109 _ _ _]
      tunnel: w311 -> [w369 w379 w388 w405 w421 w514 w611 w709 w807 w905 w1003 w1118 w1142 w1192 w1212]
      tunnel: [w369 w379 w388 w404 w419 w512 w609 w707 w805 w903 w1001 w1088 w1142 w1192 w1204] -> w349
      tunnel: w318 -> [_ _ _ _ _ _ _ _ _ _ _ _ _ _ _]
      tunnel: w345 -> [w368 w378 w387 w397 w439 w532 w629 w727 w825 w923 w1021 w1120 w1151 w1191 w1211]
      tunnel: [w367 w377 w386 w396 w416 w509 w606 w704 w802 w900 w998 w1093 w1150 w1190 w1209] -> w335
      tunnel: w344 -> [_ _ _ _ w434 w527 w624 w722 w820 w918 w1016 _ _ _ _]
      tunnel: w343 -> [_ _ _ _ w433 w526 w623 w721 w819 w917 w1015 _ _ _ _]
      tunnel: w342 -> [w367 w377 w386 w396 w417 w510 w607 w705 w803 w901 w999 w1119 w1150 w1190 w1209]
      tunnel: [w368 w378 w387 w397 w422 w515 w612 w710 w808 w906 w1004 w1114 w1151 w1191 w1210] -> w341
      tunnel: w340 -> [w366 w376 w385 w395 w430 w523 w620 w718 w816 w914 w1012 w1111 w1149 w1189 w1208]
      tunnel: [w366 w376 w385 w395 w430 w523 w620 w718 w816 w914 w1012 w1110 w1149 w1189 w1208] -> w334
      tunnel: [w365 w375 w384 w394 w418 w511 w608 w706 w804 w902 w1000 w1105 w1148 w1188 w1207] -> w339
      tunnel: w338 -> [w365 w375 w384 w394 _ _ _ _ _ _ _ w1106 w1148 w1188 w1207]
      tunnel: w336 -> [_ _ _ _ _ _ _ _ _ _ _ w1113 _ _ _]
      tunnel: w333 -> [_ _ _ _ _ _ _ _ _ _ _ w1112 _ _ _]
      tunnel: w329 -> [_ _ _ _ _ _ _ _ _ _ _ w1108 _ _ _]
      tunnel: w328 -> [w364 w374 w383 w393 w415 w508 w605 w703 w801 w899 w997 w1092 w1147 w1187 w1206]
      tunnel: [w364 w374 w383 w393 w414 w507 w604 w702 w800 w898 w996 w1092 w1147 w1187 w1206] -> w327
      tunnel: [w363 w373 w382 w392 w413 w506 w603 w701 w799 w897 w995 w1091 w1146 w1186 w1205] -> w326
      tunnel: w325 -> [w363 w373 w382 w392 w412 w505 w602 w700 w798 w896 w994 w1091 w1146 w1186 w1205]
      tunnel: w324 -> [_ _ _ _ w411 w504 w601 w699 w797 w895 w993 _ _ _ _]
      tunnel: w323 -> [w362 w372 w381 w391 w409 w502 w599 w697 w795 w893 w991 w1090 _ w1184 w1199]
      tunnel: [w361 w371 w380 w390 w410 w503 w600 w698 w796 w894 w992 w1089 w1140 _ w1200] -> w322
      tunnel: w321 -> [w361 w371 w380 w390 w410 w503 w600 w698 w796 w894 w992 w1089 w1143 w1183 w1203]
      tunnel: [_ _ _ _ _ _ _ _ _ _ _ _ FALSE ("aborted?") FALSE ("aborted?") w1202] -> w320
      tunnel: [w362 w372 w381 w391 w409 w502 w599 w697 w795 w893 w991 w1090 w1144 w1181 w1199] -> w317
      frame "TimeOut", Default {
      }
      frame "Sample Not Collected" {
        n123 = local write "Tab Control"(T3."Recording Reason Sonde" ("Tab Control")) -> ()
      }
      frame "Record Reason" {
        n124 = flat-sequence {
          frame #0 {
            n125 = local write "Tab Control"(T3."Recording Reason Sonde" ("Tab Control")) -> ()
          }
        }
      }
      frame "Continuous  Data" {
        n126 = local read "Found Quanta Sonde Com Port"() -> (w402:refnum<visa-resource-name>)
        n127 = control-ref of="Sonde Data Display"() -> (w406:refnum<vi>)
        n128 = local read "Sample Sheet Data Row Cluster 2"() -> (w398:T1)
        n129 = call "SDI-12 Continuous Operations.vi"("RS232 Port In"=w402, "Sensor Address In"="0", "Sonde Data Ctl Refnum"=w406, "Error In (No Error)"=w405) -> ("output cluster"=w403:T2, "Temperature"=w400:cluster{"Y":dbl[], "Y":dbl[]}[], "Sonde Data Display"=w399:T8, "Error Out"=w404:errorcluster)  [unwired: 8 in, 4 out]
        n130 = Bundle By Name(cluster=w398, "Sonde Data Cluster"=w403) -> (w401:T1)
        n131 = local write "Temperature"(w400) -> ()
        n132 = local write "Sonde Data Display"(w399) -> ()
        n133 = local write "Sample Sheet Data Row Cluster 2"(w401) -> ()
      }
      frame "Acq. Single Point" {
        n134 = invoke on="Record Single Sample" class="Bool" method="Reinit To Default"(error in=w421) -> (error out=w420:errorcluster)  [unwired: 2 in, 2 out]
        n135 = call <vilib>:"Clear Errors.vi"("error in (no error)"=w420) -> ("error out"=w408:errorcluster)  [unwired: 5 in, 1 out]
        n136 = call "get sample sheet data cells.vi"("error in (no error)"=w408, "NI_report in"=w439) -> ("error out"=w436:errorcluster, "data"=w438:string[][], "NI_report out"=w431:refnum<class "NI_report.lvclass">, "left edge output cluster"=w437:cluster{"row":i32, "column":i32})  [unwired: 5 in, 1 out]
        n137 = flat-sequence {
          tunnel: w436 -> [w500]
          tunnel: [w492] -> _
          tunnel: w437 -> [w498]
          tunnel: [w497] -> w435
          tunnel: [w496] -> _
          tunnel: [w495] -> w429
          tunnel: w438 -> [w492]
          frame #0 {
            n138 = Array Subset(array=w492, index (col)=2 ("index")) -> (w494:string[][])  [unwired: 3 in]
            n139 = local write "Sonde Data Array"(w494) -> ()
            n140 = local read "Current Sample Sheet"() -> (w491:string)
            n141 = call "find last occupied cell.vi"("data"=w492, "Active Sheet"=w491, "Header Rows to remove"=3, "sub array start"=w498, "error in (no error)"=w500) -> ("row max value"=w496:i32, "column max value"=w490:i32, 13:"start of last occupied row"=w495:cluster{"row":i32, "column":i32}, 14:"start of last occupied row"=w489:string, "error out"=w497:errorcluster)  [unwired: 4 in, 2 out]
            n142 = local write "last occupied cell's name"(w489) -> ()
            n143 = local write "row max value"(w490) -> ()
          }
        }
        n144 = local read "Found Quanta Sonde Com Port"() -> (w425:refnum<visa-resource-name>)
        n145 = Equal?(x=w425, y=refnum<visa-resource-name> refnum ("RS232 Port Out")) -> (x = y?=w427:bool)
        n146 = case shown="False" w427 {
          tunnel: w425 -> [w468 _]
          tunnel: [w459 w485] -> w428
          tunnel: w435 -> [w463 w488]
          tunnel: [w462 w488] -> w432
          tunnel: w415 -> [w458 w487]
          tunnel: [w457 w475] -> w414
          tunnel: [w456 w474] -> w413
          tunnel: w412 -> [w455 w486]
          tunnel: w411 -> [_ w471]
          frame False {
            n147 = control-ref of="Sonde Data Display"() -> (w464:refnum<vi>)
            n148 = local read "Sample Sheet Data Row Cluster 2"() -> (w460:T1)
            n149 = call "SDI-12 Single Operation with output cluster.vi"("RS232 Port In"=w468, "Sensor Address In"="0", "Sonde Data Ctl Refnum"=w464, "Error In (No Error)"=w463, "Time Array In"=w458, "Measurement Array In"=w455) -> ("time array out"=w457:dbl[], "Measurement  array Out"=w456:dbl[][], "output cluster"=w461:T2, "Temperature"=w466:cluster{"Y":dbl[], "Y":dbl[]}[], "Sonde Data Display"=w465:T8, "Error Out"=w462:errorcluster)  [unwired: 12 in, 4 out]
            n150 = local write "Temperature"(w466) -> ()
            n151 = local write "Sonde Data Display"(w465) -> ()
            n152 = Bundle By Name(cluster=w460, "Sonde Data Cluster"=w461) -> (w459:T1)
          }
          frame True {
            n153 = Get Date/Time In Seconds() -> (seconds since 1Jan1904=w477:timestamp)
            n154 = To Double Precision Float(number=w477) -> (double precision float=w476:dbl)
            n155 = Subtract(x=w476, y=w471) -> (x-y=w469:dbl)
            n156 = local read "Sample Sheet Data Row Cluster 2"() -> (w485:T1)
            n157 = local write "Current Time (s)"(w469) -> ()
            n158 = Unbundle By Name(w485) -> ("Sonde Data Cluster.Temp"=w470:dbl, "Sonde Data Cluster.pH"=w484:dbl, "Sonde Data Cluster.Specific\nConductance"=w483:dbl, "Sonde Data Cluster.Salinity"=w482:dbl, "Sonde Data Cluster.Dissolved\nOxygen"=w481:dbl, "Sonde Data Cluster.ORP"=w480:dbl)  [unwired: 1 out]
            n159 = Build Array(w470, w484, w483, w482, w481, 0.0 ("element"), w480) -> (w478:dbl[])
            n160 = Build Array (concatenate)(w487, w469) -> (w475:dbl[])
            n161 = Build Array (concatenate)(w486, w478) -> (w474:dbl[][])
            n162 = call "format into Sonde Vertical Graph Data Input.vi"("Sonde Measurement Array"=w474, "Time Array"=w475) -> ("Sonde Data Display"=w473:T8, "Temperature"=w472:cluster{"X":dbl[], "Y":dbl[]}[])  [unwired: 8 in]
            n163 = local write "Temperature"(w472) -> ()
            n164 = local write "Sonde Data Display"(w473) -> ()
          }
        }
        n165 = local write "Sample Sheet Data Row Cluster 2"(w428) -> ()
        n166 = call "write out sonde row.vi"("NI_report in"=w431, "Columns"=w434, "Column of Volume"=w433, "Sample Sheet Data Row Cluster"=w428, "row index"=w417, "error in (no error)"=w432, "start of last occupied row"=w429) -> ("NI_report out"=w423:refnum<class "NI_report.lvclass">, "row index out"=w416:i32, "error out"=w424:errorcluster)  [unwired: 6 in]
        n167 = flat-sequence {
          tunnel: w424 -> [w454]
          tunnel: w423 -> [w453]
          tunnel: [w452] -> w422
          tunnel: [w446] -> w419
          tunnel: [w444] -> w418
          frame #0 {
            (unwired) 3 ("Header Rows to remove")
            n168 = call <vilib>:"Clear Errors.vi"("error in (no error)"=w454) -> ("error out"=w440:errorcluster)  [unwired: 5 in, 1 out]
            n169 = local read "Current Sample Sheet"() -> (w442:string)
            n170 = call "get sample sheet data cells.vi"("error in (no error)"=w440, "NI_report in"=w453) -> ("error out"=w447:errorcluster, "data"=w448:string[][], "NI_report out"=w452:refnum<class "NI_report.lvclass">, "left edge output cluster"=w445:cluster{"row":i32, "column":i32})  [unwired: 5 in, 1 out]
            n171 = call "find last occupied cell.vi"("data"=w448, "Active Sheet"=w442, "Header Rows to remove"=3, "sub array start"=w445, "error in (no error)"=w447) -> ("row max value"=w443:i32, 13:"start of last occupied row"=w444:cluster{"row":i32, "column":i32}, 14:"start of last occupied row"=w441:string, "error out"=w446:errorcluster)  [unwired: 4 in, 3 out]
            n172 = Array Subset(array=w448, index (col)=2 ("index")) -> (w450:string[][])  [unwired: 3 in]
            n173 = local write "Sonde Data Array"(w450) -> ()
            n174 = local write "row max value"(w443) -> ()
            n175 = local write "last occupied cell's name"(w441) -> ()
          }
        }
      }
      frame "pH Calibration Zero" {
        n176 = invoke on="Record Single Sample" class="Bool" method="Reinit To Default"(error in=w514) -> (error out=w513:errorcluster)  [unwired: 2 in, 2 out]
        n177 = call <vilib>:"Clear Errors.vi"("error in (no error)"=w513) -> ("error out"=w501:errorcluster)  [unwired: 5 in, 1 out]
        n178 = call "get sample sheet data cells.vi"("error in (no error)"=w501, "NI_report in"=w532) -> ("error out"=w529:errorcluster, "data"=w531:string[][], "NI_report out"=w524:refnum<class "NI_report.lvclass">, "left edge output cluster"=w530:cluster{"row":i32, "column":i32})  [unwired: 5 in, 1 out]
        n179 = flat-sequence {
          tunnel: w529 -> [w597]
          tunnel: [w589] -> _
          tunnel: w530 -> [w595]
          tunnel: [w594] -> w528
          tunnel: [w593] -> _
          tunnel: [w592] -> w522
          tunnel: w531 -> [w589]
          frame #0 {
            n180 = Array Subset(array=w589, index (col)=2 ("index")) -> (w591:string[][])  [unwired: 3 in]
            n181 = local write "Sonde Data Array"(w591) -> ()
            n182 = local read "Current Sample Sheet"() -> (w588:string)
            n183 = call "find last occupied cell.vi"("data"=w589, "Active Sheet"=w588, "Header Rows to remove"=3, "sub array start"=w595, "error in (no error)"=w597) -> ("row max value"=w593:i32, "column max value"=w587:i32, 13:"start of last occupied row"=w592:cluster{"row":i32, "column":i32}, 14:"start of last occupied row"=w586:string, "error out"=w594:errorcluster)  [unwired: 4 in, 2 out]
            n184 = local write "last occupied cell's name"(w586) -> ()
            n185 = local write "row max value"(w587) -> ()
          }
        }
        n186 = local read "Found Quanta Sonde Com Port"() -> (w518:refnum<visa-resource-name>)
        n187 = Equal?(x=w518, y=refnum<visa-resource-name> refnum ("RS232 Port Out")) -> (x = y?=w520:bool)
        n188 = case shown="False" w520 {
          tunnel: w518 -> [w551 _]
          tunnel: [w559 w582] -> w521
          tunnel: w528 -> [w553 w585]
          tunnel: [w562 w585] -> w525
          tunnel: w508 -> [w558 w584]
          tunnel: [w557 w572] -> w507
          tunnel: [w556 w571] -> w506
          tunnel: w505 -> [w555 w583]
          tunnel: w504 -> [_ w568]
          frame False {
            w554 = "0" ("Sensor Address In")
            n189 = control-ref of="Sonde Data Display"() -> (w563:refnum<vi>)
            n190 = call "Calibrate pH Sensor.vi"("Calibration Standard"="pH Zero", "Error In (No Error)"=w553, "Sensor Address In"=w554, "RS232 Port In"=w551) -> ("Error Out"=w552:errorcluster, "Sensor Calibrate Response"=→"pH Zero \nCalibrate Response":bool, "RS232 Port Out"=w550:refnum<visa-resource-name>)  [unwired: 4 in, 1 out]
            n191 = local read "Sample Sheet Data Row Cluster 2"() -> (w560:T1)
            n192 = call "SDI-12 Single Operation with output cluster.vi"("RS232 Port In"=w550, "Sensor Address In"=w554, "Sonde Data Ctl Refnum"=w563, "Error In (No Error)"=w552, "Time Array In"=w558, "Measurement Array In"=w555) -> ("time array out"=w557:dbl[], "Measurement  array Out"=w556:dbl[][], "output cluster"=w561:T2, "Temperature"=w565:cluster{"Y":dbl[], "Y":dbl[]}[], "Sonde Data Display"=w564:T8, "Error Out"=w562:errorcluster)  [unwired: 12 in, 4 out]
            n193 = local write "Temperature"(w565) -> ()
            n194 = local write "Sonde Data Display"(w564) -> ()
            n195 = Bundle By Name(cluster=w560, "Sonde Data Cluster"=w561) -> (w559:T1)
          }
          frame True {
            n196 = Get Date/Time In Seconds() -> (seconds since 1Jan1904=w574:timestamp)
            n197 = To Double Precision Float(number=w574) -> (double precision float=w573:dbl)
            n198 = Subtract(x=w573, y=w568) -> (x-y=w566:dbl)
            n199 = local read "Sample Sheet Data Row Cluster 2"() -> (w582:T1)
            n200 = local write "Current Time (s)"(w566) -> ()
            n201 = Unbundle By Name(w582) -> ("Sonde Data Cluster.Temp"=w567:dbl, "Sonde Data Cluster.pH"=w581:dbl, "Sonde Data Cluster.Specific\nConductance"=w580:dbl, "Sonde Data Cluster.Salinity"=w579:dbl, "Sonde Data Cluster.Dissolved\nOxygen"=w578:dbl, "Sonde Data Cluster.ORP"=w577:dbl)  [unwired: 1 out]
            n202 = Build Array(w567, w581, w580, w579, w578, 0.0 ("element"), w577) -> (w575:dbl[])
            n203 = Build Array (concatenate)(w584, w566) -> (w572:dbl[])
            n204 = Build Array (concatenate)(w583, w575) -> (w571:dbl[][])
            n205 = call "format into Sonde Vertical Graph Data Input.vi"("Sonde Measurement Array"=w571, "Time Array"=w572) -> ("Sonde Data Display"=w570:T8, "Temperature"=w569:cluster{"X":dbl[], "Y":dbl[]}[])  [unwired: 8 in]
            n206 = local write "Temperature"(w569) -> ()
            n207 = local write "Sonde Data Display"(w570) -> ()
          }
        }
        n208 = local write "Sample Sheet Data Row Cluster 2"(w521) -> ()
        n209 = call "write out sonde row.vi"("NI_report in"=w524, "Columns"=w527, "Column of Volume"=w526, "Sample Sheet Data Row Cluster"=w521, "row index"=w510, "error in (no error)"=w525, "start of last occupied row"=w522) -> ("NI_report out"=w516:refnum<class "NI_report.lvclass">, "row index out"=w509:i32, "error out"=w517:errorcluster)  [unwired: 6 in]
        n210 = flat-sequence {
          tunnel: w517 -> [w547]
          tunnel: w516 -> [w546]
          tunnel: [w545] -> w515
          tunnel: [w539] -> w512
          tunnel: [w537] -> w511
          frame #0 {
            (unwired) 3 ("Header Rows to remove")
            n211 = call <vilib>:"Clear Errors.vi"("error in (no error)"=w547) -> ("error out"=w533:errorcluster)  [unwired: 5 in, 1 out]
            n212 = local read "Current Sample Sheet"() -> (w535:string)
            n213 = call "get sample sheet data cells.vi"("error in (no error)"=w533, "NI_report in"=w546) -> ("error out"=w540:errorcluster, "data"=w541:string[][], "NI_report out"=w545:refnum<class "NI_report.lvclass">, "left edge output cluster"=w538:cluster{"row":i32, "column":i32})  [unwired: 5 in, 1 out]
            n214 = call "find last occupied cell.vi"("data"=w541, "Active Sheet"=w535, "Header Rows to remove"=3, "sub array start"=w538, "error in (no error)"=w540) -> ("row max value"=w536:i32, 13:"start of last occupied row"=w537:cluster{"row":i32, "column":i32}, 14:"start of last occupied row"=w534:string, "error out"=w539:errorcluster)  [unwired: 4 in, 3 out]
            n215 = Array Subset(array=w541, index (col)=2 ("index")) -> (w543:string[][])  [unwired: 3 in]
            n216 = local write "Sonde Data Array"(w543) -> ()
            n217 = local write "row max value"(w536) -> ()
            n218 = local write "last occupied cell's name"(w534) -> ()
          }
        }
      }
      frame "pH Calibration Standard" {
        n219 = invoke on="Record Single Sample" class="Bool" method="Reinit To Default"(error in=w611) -> (error out=w610:errorcluster)  [unwired: 2 in, 2 out]
        n220 = call <vilib>:"Clear Errors.vi"("error in (no error)"=w610) -> ("error out"=w598:errorcluster)  [unwired: 5 in, 1 out]
        n221 = call "get sample sheet data cells.vi"("error in (no error)"=w598, "NI_report in"=w629) -> ("error out"=w626:errorcluster, "data"=w628:string[][], "NI_report out"=w621:refnum<class "NI_report.lvclass">, "left edge output cluster"=w627:cluster{"row":i32, "column":i32})  [unwired: 5 in, 1 out]
        n222 = flat-sequence {
          tunnel: w626 -> [w695]
          tunnel: [w687] -> _
          tunnel: w627 -> [w693]
          tunnel: [w692] -> w625
          tunnel: [w691] -> _
          tunnel: [w690] -> w619
          tunnel: w628 -> [w687]
          frame #0 {
            n223 = Array Subset(array=w687, index (col)=2 ("index")) -> (w689:string[][])  [unwired: 3 in]
            n224 = local write "Sonde Data Array"(w689) -> ()
            n225 = local read "Current Sample Sheet"() -> (w686:string)
            n226 = call "find last occupied cell.vi"("data"=w687, "Active Sheet"=w686, "Header Rows to remove"=3, "sub array start"=w693, "error in (no error)"=w695) -> ("row max value"=w691:i32, "column max value"=w685:i32, 13:"start of last occupied row"=w690:cluster{"row":i32, "column":i32}, 14:"start of last occupied row"=w684:string, "error out"=w692:errorcluster)  [unwired: 4 in, 2 out]
            n227 = local write "last occupied cell's name"(w684) -> ()
            n228 = local write "row max value"(w685) -> ()
          }
        }
        n229 = local read "Found Quanta Sonde Com Port"() -> (w615:refnum<visa-resource-name>)
        n230 = Equal?(x=w615, y=refnum<visa-resource-name> refnum ("RS232 Port Out")) -> (x = y?=w617:bool)
        n231 = case shown="False" w617 {
          tunnel: w615 -> [w646 _]
          tunnel: [w656 w680] -> w618
          tunnel: w625 -> [w649 w683]
          tunnel: [w659 w683] -> w622
          tunnel: w605 -> [w655 w682]
          tunnel: [w654 w670] -> w604
          tunnel: [w653 w669] -> w603
          tunnel: w602 -> [w652 w681]
          tunnel: w601 -> [_ w666]
          frame False {
            n232 = control-ref of="Sonde Data Display"() -> (w660:refnum<vi>)
            n233 = call "Calibrate pH Sensor.vi"("Calibration Standard"="pH Reference", "Error In (No Error)"=w649, "Sensor Address In"="0", "RS232 Port In"=w646) -> ("Error Out"=w648:errorcluster, "Sensor Calibrate Response"=→"pH  Reference\nCalibrate Response":bool, "RS232 Port Out"=w645:refnum<visa-resource-name>)  [unwired: 4 in, 1 out]
            n234 = local read "Sample Sheet Data Row Cluster 2"() -> (w657:T1)
            n235 = call "SDI-12 Single Operation with output cluster.vi"("RS232 Port In"=w645, "Sensor Address In"="0", "Sonde Data Ctl Refnum"=w660, "Error In (No Error)"=w648, "Time Array In"=w655, "Measurement Array In"=w652) -> ("time array out"=w654:dbl[], "Measurement  array Out"=w653:dbl[][], "output cluster"=w658:T2, "Temperature"=w662:cluster{"Y":dbl[], "Y":dbl[]}[], "Sonde Data Display"=w661:T8, "Error Out"=w659:errorcluster)  [unwired: 12 in, 4 out]
            n236 = local write "Temperature"(w662) -> ()
            n237 = local write "Sonde Data Display"(w661) -> ()
            n238 = Bundle By Name(cluster=w657, "Sonde Data Cluster"=w658) -> (w656:T1)
          }
          frame True {
            n239 = Get Date/Time In Seconds() -> (seconds since 1Jan1904=w672:timestamp)
            n240 = To Double Precision Float(number=w672) -> (double precision float=w671:dbl)
            n241 = Subtract(x=w671, y=w666) -> (x-y=w664:dbl)
            n242 = local read "Sample Sheet Data Row Cluster 2"() -> (w680:T1)
            n243 = local write "Current Time (s)"(w664) -> ()
            n244 = Unbundle By Name(w680) -> ("Sonde Data Cluster.Temp"=w665:dbl, "Sonde Data Cluster.pH"=w679:dbl, "Sonde Data Cluster.Specific\nConductance"=w678:dbl, "Sonde Data Cluster.Salinity"=w677:dbl, "Sonde Data Cluster.Dissolved\nOxygen"=w676:dbl, "Sonde Data Cluster.ORP"=w675:dbl)  [unwired: 1 out]
            n245 = Build Array(w665, w679, w678, w677, w676, 0.0 ("element"), w675) -> (w673:dbl[])
            n246 = Build Array (concatenate)(w682, w664) -> (w670:dbl[])
            n247 = Build Array (concatenate)(w681, w673) -> (w669:dbl[][])
            n248 = call "format into Sonde Vertical Graph Data Input.vi"("Sonde Measurement Array"=w669, "Time Array"=w670) -> ("Sonde Data Display"=w668:T8, "Temperature"=w667:cluster{"X":dbl[], "Y":dbl[]}[])  [unwired: 8 in]
            n249 = local write "Temperature"(w667) -> ()
            n250 = local write "Sonde Data Display"(w668) -> ()
          }
        }
        n251 = local write "Sample Sheet Data Row Cluster 2"(w618) -> ()
        n252 = call "write out sonde row.vi"("NI_report in"=w621, "Columns"=w624, "Column of Volume"=w623, "Sample Sheet Data Row Cluster"=w618, "row index"=w607, "error in (no error)"=w622, "start of last occupied row"=w619) -> ("NI_report out"=w613:refnum<class "NI_report.lvclass">, "row index out"=w606:i32, "error out"=w614:errorcluster)  [unwired: 6 in]
        n253 = flat-sequence {
          tunnel: w614 -> [w644]
          tunnel: w613 -> [w643]
          tunnel: [w642] -> w612
          tunnel: [w636] -> w609
          tunnel: [w634] -> w608
          frame #0 {
            (unwired) 3 ("Header Rows to remove")
            n254 = call <vilib>:"Clear Errors.vi"("error in (no error)"=w644) -> ("error out"=w630:errorcluster)  [unwired: 5 in, 1 out]
            n255 = local read "Current Sample Sheet"() -> (w632:string)
            n256 = call "get sample sheet data cells.vi"("error in (no error)"=w630, "NI_report in"=w643) -> ("error out"=w637:errorcluster, "data"=w638:string[][], "NI_report out"=w642:refnum<class "NI_report.lvclass">, "left edge output cluster"=w635:cluster{"row":i32, "column":i32})  [unwired: 5 in, 1 out]
            n257 = call "find last occupied cell.vi"("data"=w638, "Active Sheet"=w632, "Header Rows to remove"=3, "sub array start"=w635, "error in (no error)"=w637) -> ("row max value"=w633:i32, 13:"start of last occupied row"=w634:cluster{"row":i32, "column":i32}, 14:"start of last occupied row"=w631:string, "error out"=w636:errorcluster)  [unwired: 4 in, 3 out]
            n258 = Array Subset(array=w638, index (col)=2 ("index")) -> (w640:string[][])  [unwired: 3 in]
            n259 = local write "Sonde Data Array"(w640) -> ()
            n260 = local write "row max value"(w633) -> ()
            n261 = local write "last occupied cell's name"(w631) -> ()
          }
        }
      }
      frame "ORP Calibration Standard" {
        n262 = invoke on="Record Single Sample" class="Bool" method="Reinit To Default"(error in=w709) -> (error out=w708:errorcluster)  [unwired: 2 in, 2 out]
        n263 = call <vilib>:"Clear Errors.vi"("error in (no error)"=w708) -> ("error out"=w696:errorcluster)  [unwired: 5 in, 1 out]
        n264 = call "get sample sheet data cells.vi"("error in (no error)"=w696, "NI_report in"=w727) -> ("error out"=w724:errorcluster, "data"=w726:string[][], "NI_report out"=w719:refnum<class "NI_report.lvclass">, "left edge output cluster"=w725:cluster{"row":i32, "column":i32})  [unwired: 5 in, 1 out]
        n265 = flat-sequence {
          tunnel: w724 -> [w793]
          tunnel: [w785] -> _
          tunnel: w725 -> [w791]
          tunnel: [w790] -> w723
          tunnel: [w789] -> _
          tunnel: [w788] -> w717
          tunnel: w726 -> [w785]
          frame #0 {
            n266 = Array Subset(array=w785, index (col)=2 ("index")) -> (w787:string[][])  [unwired: 3 in]
            n267 = local write "Sonde Data Array"(w787) -> ()
            n268 = local read "Current Sample Sheet"() -> (w784:string)
            n269 = call "find last occupied cell.vi"("data"=w785, "Active Sheet"=w784, "Header Rows to remove"=3, "sub array start"=w791, "error in (no error)"=w793) -> ("row max value"=w789:i32, "column max value"=w783:i32, 13:"start of last occupied row"=w788:cluster{"row":i32, "column":i32}, 14:"start of last occupied row"=w782:string, "error out"=w790:errorcluster)  [unwired: 4 in, 2 out]
            n270 = local write "last occupied cell's name"(w782) -> ()
            n271 = local write "row max value"(w783) -> ()
          }
        }
        n272 = local read "Found Quanta Sonde Com Port"() -> (w713:refnum<visa-resource-name>)
        n273 = Equal?(x=w713, y=refnum<visa-resource-name> refnum ("RS232 Port Out")) -> (x = y?=w715:bool)
        n274 = case shown="False" w715 {
          tunnel: w713 -> [w744 _]
          tunnel: [w754 w778] -> w716
          tunnel: w723 -> [w746 w781]
          tunnel: [w757 w781] -> w720
          tunnel: w703 -> [w753 w780]
          tunnel: [w752 w768] -> w702
          tunnel: [w751 w767] -> w701
          tunnel: w700 -> [w750 w779]
          tunnel: w699 -> [_ w764]
          frame False {
            n275 = control-ref of="Sonde Data Display"() -> (w758:refnum<vi>)
            n276 = call "Calibrate ORP Sensor.vi"("Calibration Standard"="ORP Reference", "Error In (No Error)"=w746, "Sensor Address In"="0", "RS232 Port In"=w744) -> ("Error Out"=w745:errorcluster, "Sensor Calibrate Response"=→"ORP  Reference\nCalibrate Response":bool, "RS232 Port Out"=w743:refnum<visa-resource-name>)  [unwired: 4 in, 1 out]
            n277 = local read "Sample Sheet Data Row Cluster 2"() -> (w755:T1)
            n278 = call "SDI-12 Single Operation with output cluster.vi"("RS232 Port In"=w743, "Sensor Address In"="0", "Sonde Data Ctl Refnum"=w758, "Error In (No Error)"=w745, "Time Array In"=w753, "Measurement Array In"=w750) -> ("time array out"=w752:dbl[], "Measurement  array Out"=w751:dbl[][], "output cluster"=w756:T2, "Temperature"=w760:cluster{"Y":dbl[], "Y":dbl[]}[], "Sonde Data Display"=w759:T8, "Error Out"=w757:errorcluster)  [unwired: 12 in, 4 out]
            n279 = local write "Temperature"(w760) -> ()
            n280 = local write "Sonde Data Display"(w759) -> ()
            n281 = Bundle By Name(cluster=w755, "Sonde Data Cluster"=w756) -> (w754:T1)
          }
          frame True {
            n282 = Get Date/Time In Seconds() -> (seconds since 1Jan1904=w770:timestamp)
            n283 = To Double Precision Float(number=w770) -> (double precision float=w769:dbl)
            n284 = Subtract(x=w769, y=w764) -> (x-y=w762:dbl)
            n285 = local read "Sample Sheet Data Row Cluster 2"() -> (w778:T1)
            n286 = local write "Current Time (s)"(w762) -> ()
            n287 = Unbundle By Name(w778) -> ("Sonde Data Cluster.Temp"=w763:dbl, "Sonde Data Cluster.pH"=w777:dbl, "Sonde Data Cluster.Specific\nConductance"=w776:dbl, "Sonde Data Cluster.Salinity"=w775:dbl, "Sonde Data Cluster.Dissolved\nOxygen"=w774:dbl, "Sonde Data Cluster.ORP"=w773:dbl)  [unwired: 1 out]
            n288 = Build Array(w763, w777, w776, w775, w774, 0.0 ("element"), w773) -> (w771:dbl[])
            n289 = Build Array (concatenate)(w780, w762) -> (w768:dbl[])
            n290 = Build Array (concatenate)(w779, w771) -> (w767:dbl[][])
            n291 = call "format into Sonde Vertical Graph Data Input.vi"("Sonde Measurement Array"=w767, "Time Array"=w768) -> ("Sonde Data Display"=w766:T8, "Temperature"=w765:cluster{"X":dbl[], "Y":dbl[]}[])  [unwired: 8 in]
            n292 = local write "Temperature"(w765) -> ()
            n293 = local write "Sonde Data Display"(w766) -> ()
          }
        }
        n294 = local write "Sample Sheet Data Row Cluster 2"(w716) -> ()
        n295 = call "write out sonde row.vi"("NI_report in"=w719, "Columns"=w722, "Column of Volume"=w721, "Sample Sheet Data Row Cluster"=w716, "row index"=w705, "error in (no error)"=w720, "start of last occupied row"=w717) -> ("NI_report out"=w711:refnum<class "NI_report.lvclass">, "row index out"=w704:i32, "error out"=w712:errorcluster)  [unwired: 6 in]
        n296 = flat-sequence {
          tunnel: w712 -> [w742]
          tunnel: w711 -> [w741]
          tunnel: [w740] -> w710
          tunnel: [w734] -> w707
          tunnel: [w732] -> w706
          frame #0 {
            (unwired) 3 ("Header Rows to remove")
            n297 = call <vilib>:"Clear Errors.vi"("error in (no error)"=w742) -> ("error out"=w728:errorcluster)  [unwired: 5 in, 1 out]
            n298 = local read "Current Sample Sheet"() -> (w730:string)
            n299 = call "get sample sheet data cells.vi"("error in (no error)"=w728, "NI_report in"=w741) -> ("error out"=w735:errorcluster, "data"=w736:string[][], "NI_report out"=w740:refnum<class "NI_report.lvclass">, "left edge output cluster"=w733:cluster{"row":i32, "column":i32})  [unwired: 5 in, 1 out]
            n300 = call "find last occupied cell.vi"("data"=w736, "Active Sheet"=w730, "Header Rows to remove"=3, "sub array start"=w733, "error in (no error)"=w735) -> ("row max value"=w731:i32, 13:"start of last occupied row"=w732:cluster{"row":i32, "column":i32}, 14:"start of last occupied row"=w729:string, "error out"=w734:errorcluster)  [unwired: 4 in, 3 out]
            n301 = Array Subset(array=w736, index (col)=2 ("index")) -> (w738:string[][])  [unwired: 3 in]
            n302 = local write "Sonde Data Array"(w738) -> ()
            n303 = local write "row max value"(w731) -> ()
            n304 = local write "last occupied cell's name"(w729) -> ()
          }
        }
      }
      frame "Salinity Calibration Standard" {
        n305 = invoke on="Record Single Sample" class="Bool" method="Reinit To Default"(error in=w807) -> (error out=w806:errorcluster)  [unwired: 2 in, 2 out]
        n306 = call <vilib>:"Clear Errors.vi"("error in (no error)"=w806) -> ("error out"=w794:errorcluster)  [unwired: 5 in, 1 out]
        n307 = call "get sample sheet data cells.vi"("error in (no error)"=w794, "NI_report in"=w825) -> ("error out"=w822:errorcluster, "data"=w824:string[][], "NI_report out"=w817:refnum<class "NI_report.lvclass">, "left edge output cluster"=w823:cluster{"row":i32, "column":i32})  [unwired: 5 in, 1 out]
        n308 = flat-sequence {
          tunnel: w822 -> [w891]
          tunnel: [w883] -> _
          tunnel: w823 -> [w889]
          tunnel: [w888] -> w821
          tunnel: [w887] -> _
          tunnel: [w886] -> w815
          tunnel: w824 -> [w883]
          frame #0 {
            n309 = Array Subset(array=w883, index (col)=2 ("index")) -> (w885:string[][])  [unwired: 3 in]
            n310 = local write "Sonde Data Array"(w885) -> ()
            n311 = local read "Current Sample Sheet"() -> (w882:string)
            n312 = call "find last occupied cell.vi"("data"=w883, "Active Sheet"=w882, "Header Rows to remove"=3, "sub array start"=w889, "error in (no error)"=w891) -> ("row max value"=w887:i32, "column max value"=w881:i32, 13:"start of last occupied row"=w886:cluster{"row":i32, "column":i32}, 14:"start of last occupied row"=w880:string, "error out"=w888:errorcluster)  [unwired: 4 in, 2 out]
            n313 = local write "last occupied cell's name"(w880) -> ()
            n314 = local write "row max value"(w881) -> ()
          }
        }
        n315 = local read "Found Quanta Sonde Com Port"() -> (w811:refnum<visa-resource-name>)
        n316 = Equal?(x=w811, y=refnum<visa-resource-name> refnum ("RS232 Port Out")) -> (x = y?=w813:bool)
        n317 = case shown="False" w813 {
          tunnel: w811 -> [w845 _]
          tunnel: [w852 w876] -> w814
          tunnel: w821 -> [w843 w879]
          tunnel: [w855 w879] -> w818
          tunnel: w801 -> [w851 w878]
          tunnel: [w850 w866] -> w800
          tunnel: [w849 w865] -> w799
          tunnel: w798 -> [w848 w877]
          tunnel: w797 -> [_ w862]
          frame False {
            n318 = call "Calibrate Salinity Sensor.vi"("Calibration Standard"="Salinity \nReference", "Error In (No Error)"=w843, "Sensor Address In"="0", "RS232 Port In"=w845) -> ("Error Out"=w842:errorcluster, "Sensor Calibrate Response"=→"Salinity  Reference\nCalibrate Response":bool, "RS232 Port Out"=w844:refnum<visa-resource-name>)  [unwired: 4 in, 1 out]
            n319 = control-ref of="Sonde Data Display"() -> (w856:refnum<vi>)
            n320 = local read "Sample Sheet Data Row Cluster 2"() -> (w853:T1)
            n321 = call "SDI-12 Single Operation with output cluster.vi"("RS232 Port In"=w844, "Sensor Address In"="0", "Sonde Data Ctl Refnum"=w856, "Error In (No Error)"=w842, "Time Array In"=w851, "Measurement Array In"=w848) -> ("time array out"=w850:dbl[], "Measurement  array Out"=w849:dbl[][], "output cluster"=w854:T2, "Temperature"=w858:cluster{"Y":dbl[], "Y":dbl[]}[], "Sonde Data Display"=w857:T8, "Error Out"=w855:errorcluster)  [unwired: 12 in, 4 out]
            n322 = local write "Temperature"(w858) -> ()
            n323 = local write "Sonde Data Display"(w857) -> ()
            n324 = Bundle By Name(cluster=w853, "Sonde Data Cluster"=w854) -> (w852:T1)
          }
          frame True {
            n325 = Get Date/Time In Seconds() -> (seconds since 1Jan1904=w868:timestamp)
            n326 = To Double Precision Float(number=w868) -> (double precision float=w867:dbl)
            n327 = Subtract(x=w867, y=w862) -> (x-y=w860:dbl)
            n328 = local read "Sample Sheet Data Row Cluster 2"() -> (w876:T1)
            n329 = local write "Current Time (s)"(w860) -> ()
            n330 = Unbundle By Name(w876) -> ("Sonde Data Cluster.Temp"=w861:dbl, "Sonde Data Cluster.pH"=w875:dbl, "Sonde Data Cluster.Specific\nConductance"=w874:dbl, "Sonde Data Cluster.Salinity"=w873:dbl, "Sonde Data Cluster.Dissolved\nOxygen"=w872:dbl, "Sonde Data Cluster.ORP"=w871:dbl)  [unwired: 1 out]
            n331 = Build Array(w861, w875, w874, w873, w872, 0.0 ("element"), w871) -> (w869:dbl[])
            n332 = Build Array (concatenate)(w878, w860) -> (w866:dbl[])
            n333 = Build Array (concatenate)(w877, w869) -> (w865:dbl[][])
            n334 = call "format into Sonde Vertical Graph Data Input.vi"("Sonde Measurement Array"=w865, "Time Array"=w866) -> ("Sonde Data Display"=w864:T8, "Temperature"=w863:cluster{"X":dbl[], "Y":dbl[]}[])  [unwired: 8 in]
            n335 = local write "Temperature"(w863) -> ()
            n336 = local write "Sonde Data Display"(w864) -> ()
          }
        }
        n337 = local write "Sample Sheet Data Row Cluster 2"(w814) -> ()
        n338 = call "write out sonde row.vi"("NI_report in"=w817, "Columns"=w820, "Column of Volume"=w819, "Sample Sheet Data Row Cluster"=w814, "row index"=w803, "error in (no error)"=w818, "start of last occupied row"=w815) -> ("NI_report out"=w809:refnum<class "NI_report.lvclass">, "row index out"=w802:i32, "error out"=w810:errorcluster)  [unwired: 6 in]
        n339 = flat-sequence {
          tunnel: w810 -> [w840]
          tunnel: w809 -> [w839]
          tunnel: [w838] -> w808
          tunnel: [w832] -> w805
          tunnel: [w830] -> w804
          frame #0 {
            (unwired) 3 ("Header Rows to remove")
            n340 = call <vilib>:"Clear Errors.vi"("error in (no error)"=w840) -> ("error out"=w826:errorcluster)  [unwired: 5 in, 1 out]
            n341 = local read "Current Sample Sheet"() -> (w828:string)
            n342 = call "get sample sheet data cells.vi"("error in (no error)"=w826, "NI_report in"=w839) -> ("error out"=w833:errorcluster, "data"=w834:string[][], "NI_report out"=w838:refnum<class "NI_report.lvclass">, "left edge output cluster"=w831:cluster{"row":i32, "column":i32})  [unwired: 5 in, 1 out]
            n343 = call "find last occupied cell.vi"("data"=w834, "Active Sheet"=w828, "Header Rows to remove"=3, "sub array start"=w831, "error in (no error)"=w833) -> ("row max value"=w829:i32, 13:"start of last occupied row"=w830:cluster{"row":i32, "column":i32}, 14:"start of last occupied row"=w827:string, "error out"=w832:errorcluster)  [unwired: 4 in, 3 out]
            n344 = Array Subset(array=w834, index (col)=2 ("index")) -> (w836:string[][])  [unwired: 3 in]
            n345 = local write "Sonde Data Array"(w836) -> ()
            n346 = local write "row max value"(w829) -> ()
            n347 = local write "last occupied cell's name"(w827) -> ()
          }
        }
      }
      frame "DO Calibration Standard" {
        n348 = invoke on="Record Single Sample" class="Bool" method="Reinit To Default"(error in=w905) -> (error out=w904:errorcluster)  [unwired: 2 in, 2 out]
        n349 = call <vilib>:"Clear Errors.vi"("error in (no error)"=w904) -> ("error out"=w892:errorcluster)  [unwired: 5 in, 1 out]
        n350 = call "get sample sheet data cells.vi"("error in (no error)"=w892, "NI_report in"=w923) -> ("error out"=w920:errorcluster, "data"=w922:string[][], "NI_report out"=w915:refnum<class "NI_report.lvclass">, "left edge output cluster"=w921:cluster{"row":i32, "column":i32})  [unwired: 5 in, 1 out]
        n351 = flat-sequence {
          tunnel: w920 -> [w989]
          tunnel: [w981] -> _
          tunnel: w921 -> [w987]
          tunnel: [w986] -> w919
          tunnel: [w985] -> _
          tunnel: [w984] -> w913
          tunnel: w922 -> [w981]
          frame #0 {
            n352 = Array Subset(array=w981, index (col)=2 ("index")) -> (w983:string[][])  [unwired: 3 in]
            n353 = local write "Sonde Data Array"(w983) -> ()
            n354 = local read "Current Sample Sheet"() -> (w980:string)
            n355 = call "find last occupied cell.vi"("data"=w981, "Active Sheet"=w980, "Header Rows to remove"=3, "sub array start"=w987, "error in (no error)"=w989) -> ("row max value"=w985:i32, "column max value"=w979:i32, 13:"start of last occupied row"=w984:cluster{"row":i32, "column":i32}, 14:"start of last occupied row"=w978:string, "error out"=w986:errorcluster)  [unwired: 4 in, 2 out]
            n356 = local write "last occupied cell's name"(w978) -> ()
            n357 = local write "row max value"(w979) -> ()
          }
        }
        n358 = local read "Found Quanta Sonde Com Port"() -> (w909:refnum<visa-resource-name>)
        n359 = Equal?(x=w909, y=refnum<visa-resource-name> refnum ("RS232 Port Out")) -> (x = y?=w911:bool)
        n360 = case shown="False" w911 {
          tunnel: w909 -> [w943 _]
          tunnel: [w950 w974] -> w912
          tunnel: w919 -> [w945 w977]
          tunnel: [w953 w977] -> w916
          tunnel: w899 -> [w949 w976]
          tunnel: [w948 w964] -> w898
          tunnel: [w947 w963] -> w897
          tunnel: w896 -> [w946 w975]
          tunnel: w895 -> [_ w960]
          frame False {
            n361 = control-ref of="Sonde Data Display"() -> (w954:refnum<vi>)
            n362 = call "Calibrate DO Sensor.vi"("Calibration Standard"="DO \nReference", "Error In (No Error)"=w945, "Sensor Address In"="0", "RS232 Port In"=w943) -> ("Error Out"=w944:errorcluster, "Sensor Calibrate Response"=→"DO  Reference\nCalibrate Response":bool, "RS232 Port Out"=w942:refnum<visa-resource-name>)  [unwired: 4 in, 1 out]
            n363 = local read "Sample Sheet Data Row Cluster 2"() -> (w951:T1)
            n364 = call "SDI-12 Single Operation with output cluster.vi"("RS232 Port In"=w942, "Sensor Address In"="0", "Sonde Data Ctl Refnum"=w954, "Error In (No Error)"=w944, "Time Array In"=w949, "Measurement Array In"=w946) -> ("time array out"=w948:dbl[], "Measurement  array Out"=w947:dbl[][], "output cluster"=w952:T2, "Temperature"=w956:cluster{"Y":dbl[], "Y":dbl[]}[], "Sonde Data Display"=w955:T8, "Error Out"=w953:errorcluster)  [unwired: 12 in, 4 out]
            n365 = local write "Temperature"(w956) -> ()
            n366 = local write "Sonde Data Display"(w955) -> ()
            n367 = Bundle By Name(cluster=w951, "Sonde Data Cluster"=w952) -> (w950:T1)
          }
          frame True {
            n368 = Get Date/Time In Seconds() -> (seconds since 1Jan1904=w966:timestamp)
            n369 = To Double Precision Float(number=w966) -> (double precision float=w965:dbl)
            n370 = Subtract(x=w965, y=w960) -> (x-y=w958:dbl)
            n371 = local read "Sample Sheet Data Row Cluster 2"() -> (w974:T1)
            n372 = local write "Current Time (s)"(w958) -> ()
            n373 = Unbundle By Name(w974) -> ("Sonde Data Cluster.Temp"=w959:dbl, "Sonde Data Cluster.pH"=w973:dbl, "Sonde Data Cluster.Specific\nConductance"=w972:dbl, "Sonde Data Cluster.Salinity"=w971:dbl, "Sonde Data Cluster.Dissolved\nOxygen"=w970:dbl, "Sonde Data Cluster.ORP"=w969:dbl)  [unwired: 1 out]
            n374 = Build Array(w959, w973, w972, w971, w970, 0.0 ("element"), w969) -> (w967:dbl[])
            n375 = Build Array (concatenate)(w976, w958) -> (w964:dbl[])
            n376 = Build Array (concatenate)(w975, w967) -> (w963:dbl[][])
            n377 = call "format into Sonde Vertical Graph Data Input.vi"("Sonde Measurement Array"=w963, "Time Array"=w964) -> ("Sonde Data Display"=w962:T8, "Temperature"=w961:cluster{"X":dbl[], "Y":dbl[]}[])  [unwired: 8 in]
            n378 = local write "Temperature"(w961) -> ()
            n379 = local write "Sonde Data Display"(w962) -> ()
          }
        }
        n380 = local write "Sample Sheet Data Row Cluster 2"(w912) -> ()
        n381 = call "write out sonde row.vi"("NI_report in"=w915, "Columns"=w918, "Column of Volume"=w917, "Sample Sheet Data Row Cluster"=w912, "row index"=w901, "error in (no error)"=w916, "start of last occupied row"=w913) -> ("NI_report out"=w907:refnum<class "NI_report.lvclass">, "row index out"=w900:i32, "error out"=w908:errorcluster)  [unwired: 6 in]
        n382 = flat-sequence {
          tunnel: w908 -> [w938]
          tunnel: w907 -> [w937]
          tunnel: [w936] -> w906
          tunnel: [w930] -> w903
          tunnel: [w928] -> w902
          frame #0 {
            (unwired) 3 ("Header Rows to remove")
            n383 = call <vilib>:"Clear Errors.vi"("error in (no error)"=w938) -> ("error out"=w924:errorcluster)  [unwired: 5 in, 1 out]
            n384 = local read "Current Sample Sheet"() -> (w926:string)
            n385 = call "get sample sheet data cells.vi"("error in (no error)"=w924, "NI_report in"=w937) -> ("error out"=w931:errorcluster, "data"=w932:string[][], "NI_report out"=w936:refnum<class "NI_report.lvclass">, "left edge output cluster"=w929:cluster{"row":i32, "column":i32})  [unwired: 5 in, 1 out]
            n386 = call "find last occupied cell.vi"("data"=w932, "Active Sheet"=w926, "Header Rows to remove"=3, "sub array start"=w929, "error in (no error)"=w931) -> ("row max value"=w927:i32, 13:"start of last occupied row"=w928:cluster{"row":i32, "column":i32}, 14:"start of last occupied row"=w925:string, "error out"=w930:errorcluster)  [unwired: 4 in, 3 out]
            n387 = Array Subset(array=w932, index (col)=2 ("index")) -> (w934:string[][])  [unwired: 3 in]
            n388 = local write "Sonde Data Array"(w934) -> ()
            n389 = local write "row max value"(w927) -> ()
            n390 = local write "last occupied cell's name"(w925) -> ()
          }
        }
      }
      frame "SC Calibration Standard" {
        n391 = invoke on="Record Single Sample" class="Bool" method="Reinit To Default"(error in=w1003) -> (error out=w1002:errorcluster)  [unwired: 2 in, 2 out]
        n392 = call <vilib>:"Clear Errors.vi"("error in (no error)"=w1002) -> ("error out"=w990:errorcluster)  [unwired: 5 in, 1 out]
        n393 = call "get sample sheet data cells.vi"("error in (no error)"=w990, "NI_report in"=w1021) -> ("error out"=w1018:errorcluster, "data"=w1020:string[][], "NI_report out"=w1013:refnum<class "NI_report.lvclass">, "left edge output cluster"=w1019:cluster{"row":i32, "column":i32})  [unwired: 5 in, 1 out]
        n394 = flat-sequence {
          tunnel: w1018 -> [w1087]
          tunnel: [w1079] -> _
          tunnel: w1019 -> [w1085]
          tunnel: [w1084] -> w1017
          tunnel: [w1083] -> _
          tunnel: [w1082] -> w1011
          tunnel: w1020 -> [w1079]
          frame #0 {
            n395 = Array Subset(array=w1079, index (col)=2 ("index")) -> (w1081:string[][])  [unwired: 3 in]
            n396 = local write "Sonde Data Array"(w1081) -> ()
            n397 = local read "Current Sample Sheet"() -> (w1078:string)
            n398 = call "find last occupied cell.vi"("data"=w1079, "Active Sheet"=w1078, "Header Rows to remove"=3, "sub array start"=w1085, "error in (no error)"=w1087) -> ("row max value"=w1083:i32, "column max value"=w1077:i32, 13:"start of last occupied row"=w1082:cluster{"row":i32, "column":i32}, 14:"start of last occupied row"=w1076:string, "error out"=w1084:errorcluster)  [unwired: 4 in, 2 out]
            n399 = local write "last occupied cell's name"(w1076) -> ()
            n400 = local write "row max value"(w1077) -> ()
          }
        }
        n401 = local read "Found Quanta Sonde Com Port"() -> (w1007:refnum<visa-resource-name>)
        n402 = Equal?(x=w1007, y=refnum<visa-resource-name> refnum ("RS232 Port Out")) -> (x = y?=w1009:bool)
        n403 = case shown="False" w1009 {
          tunnel: w1007 -> [w1042 _]
          tunnel: [w1048 w1072] -> w1010
          tunnel: w1017 -> [w1040 w1075]
          tunnel: [w1051 w1075] -> w1014
          tunnel: w997 -> [w1047 w1074]
          tunnel: [w1046 w1062] -> w996
          tunnel: [w1045 w1061] -> w995
          tunnel: w994 -> [w1044 w1073]
          tunnel: w993 -> [_ w1058]
          frame False {
            n404 = control-ref of="Sonde Data Display"() -> (w1052:refnum<vi>)
            n405 = call "Calibrate SC Sensor.vi"("Calibration Standard"="SC \nReference", "Error In (No Error)"=w1040, "Sensor Address In"="0", "RS232 Port In"=w1042) -> ("Error Out"=w1039:errorcluster, "Sensor Calibrate Response"=→"SC  Reference\nCalibrate Response":bool, "RS232 Port Out"=w1041:refnum<visa-resource-name>)  [unwired: 4 in, 1 out]
            n406 = local read "Sample Sheet Data Row Cluster 2"() -> (w1049:T1)
            n407 = call "SDI-12 Single Operation with output cluster.vi"("RS232 Port In"=w1041, "Sensor Address In"="0", "Sonde Data Ctl Refnum"=w1052, "Error In (No Error)"=w1039, "Time Array In"=w1047, "Measurement Array In"=w1044) -> ("time array out"=w1046:dbl[], "Measurement  array Out"=w1045:dbl[][], "output cluster"=w1050:T2, "Temperature"=w1054:cluster{"Y":dbl[], "Y":dbl[]}[], "Sonde Data Display"=w1053:T8, "Error Out"=w1051:errorcluster)  [unwired: 12 in, 4 out]
            n408 = local write "Temperature"(w1054) -> ()
            n409 = local write "Sonde Data Display"(w1053) -> ()
            n410 = Bundle By Name(cluster=w1049, "Sonde Data Cluster"=w1050) -> (w1048:T1)
          }
          frame True {
            n411 = Get Date/Time In Seconds() -> (seconds since 1Jan1904=w1064:timestamp)
            n412 = To Double Precision Float(number=w1064) -> (double precision float=w1063:dbl)
            n413 = Subtract(x=w1063, y=w1058) -> (x-y=w1056:dbl)
            n414 = local read "Sample Sheet Data Row Cluster 2"() -> (w1072:T1)
            n415 = local write "Current Time (s)"(w1056) -> ()
            n416 = Unbundle By Name(w1072) -> ("Sonde Data Cluster.Temp"=w1057:dbl, "Sonde Data Cluster.pH"=w1071:dbl, "Sonde Data Cluster.Specific\nConductance"=w1070:dbl, "Sonde Data Cluster.Salinity"=w1069:dbl, "Sonde Data Cluster.Dissolved\nOxygen"=w1068:dbl, "Sonde Data Cluster.ORP"=w1067:dbl)  [unwired: 1 out]
            n417 = Build Array(w1057, w1071, w1070, w1069, w1068, 0.0 ("element"), w1067) -> (w1065:dbl[])
            n418 = Build Array (concatenate)(w1074, w1056) -> (w1062:dbl[])
            n419 = Build Array (concatenate)(w1073, w1065) -> (w1061:dbl[][])
            n420 = call "format into Sonde Vertical Graph Data Input.vi"("Sonde Measurement Array"=w1061, "Time Array"=w1062) -> ("Sonde Data Display"=w1060:T8, "Temperature"=w1059:cluster{"X":dbl[], "Y":dbl[]}[])  [unwired: 8 in]
            n421 = local write "Temperature"(w1059) -> ()
            n422 = local write "Sonde Data Display"(w1060) -> ()
          }
        }
        n423 = local write "Sample Sheet Data Row Cluster 2"(w1010) -> ()
        n424 = call "write out sonde row.vi"("NI_report in"=w1013, "Columns"=w1016, "Column of Volume"=w1015, "Sample Sheet Data Row Cluster"=w1010, "row index"=w999, "error in (no error)"=w1014, "start of last occupied row"=w1011) -> ("NI_report out"=w1005:refnum<class "NI_report.lvclass">, "row index out"=w998:i32, "error out"=w1006:errorcluster)  [unwired: 6 in]
        n425 = flat-sequence {
          tunnel: w1006 -> [w1036]
          tunnel: w1005 -> [w1035]
          tunnel: [w1034] -> w1004
          tunnel: [w1028] -> w1001
          tunnel: [w1026] -> w1000
          frame #0 {
            (unwired) 3 ("Header Rows to remove")
            n426 = call <vilib>:"Clear Errors.vi"("error in (no error)"=w1036) -> ("error out"=w1022:errorcluster)  [unwired: 5 in, 1 out]
            n427 = local read "Current Sample Sheet"() -> (w1024:string)
            n428 = call "get sample sheet data cells.vi"("error in (no error)"=w1022, "NI_report in"=w1035) -> ("error out"=w1029:errorcluster, "data"=w1030:string[][], "NI_report out"=w1034:refnum<class "NI_report.lvclass">, "left edge output cluster"=w1027:cluster{"row":i32, "column":i32})  [unwired: 5 in, 1 out]
            n429 = call "find last occupied cell.vi"("data"=w1030, "Active Sheet"=w1024, "Header Rows to remove"=3, "sub array start"=w1027, "error in (no error)"=w1029) -> ("row max value"=w1025:i32, 13:"start of last occupied row"=w1026:cluster{"row":i32, "column":i32}, 14:"start of last occupied row"=w1023:string, "error out"=w1028:errorcluster)  [unwired: 4 in, 3 out]
            n430 = Array Subset(array=w1030, index (col)=2 ("index")) -> (w1032:string[][])  [unwired: 3 in]
            n431 = local write "Sonde Data Array"(w1032) -> ()
            n432 = local write "row max value"(w1025) -> ()
            n433 = local write "last occupied cell's name"(w1023) -> ()
          }
        }
      }
      frame "Write Sample Sheet" {
        n434 = Not Equal?(x=w1109, y=w1108) -> (x != y?=w1107:bool)
        n435 = Decrement(x=w1119) -> (x-1=w1093:i32)
        n436 = case shown="True" w1107 {
          tunnel: w1120 -> [w1123 w1130]
          tunnel: w1106 -> [_ w1129]
          tunnel: w1118 -> [w1122 w1128]
          tunnel: [w1122 w1127] -> w1117
          tunnel: [w1123 w1126] -> w1116
          tunnel: w1111 -> [w1121 w1125]
          tunnel: [w1121 w1124] -> w1110
          frame False {
          }
          frame True {
            n437 = flat-sequence {
              tunnel: [w1139] -> w1126
              tunnel: w1130 -> [w1138]
              tunnel: w1129 -> [w1135]
              tunnel: w1128 -> [w1134]
              tunnel: [w1133] -> w1127
              tunnel: w1125 -> [w1132]
              tunnel: [w1131] -> w1124
              frame #0 {
                n438 = Increment(x=w1132) -> (x+1=w1131:i32)
                n439 = call "write comment cell with column offset.vi"("Column Relative?"=TRUE, "comment string"="done", "error in (no error)"=w1134, "start of last occupied row"=w1135, "NI_report in"=w1138) -> ("error out"=w1133:errorcluster, "NI_report out"=w1139:refnum<class "NI_report.lvclass">)  [unwired: 5 in]
              }
            }
          }
        }
        n440 = call "open select sample sheet.vi"("Number of Sample Sheets"=w1112, "error in (no error)"=w1117, "Worksheet Names"=w1113, "Active Sample Sheet"=w1110, "NI_report in"=w1116) -> ("error out"=w1103:errorcluster, "Current Sample Sheet"=w1104:string, "NI_report out"=w1102:refnum<class "NI_report.lvclass">)  [unwired: 3 in, 1 out]
        n441 = local write "Current Sample Sheet"(w1104) -> ()
        n442 = local read "Current Sample Sheet"() -> (w1095:string)
        n443 = call "get sample sheet data cells.vi"("error in (no error)"=w1103, "NI_report in"=w1102) -> ("error out"=w1115:errorcluster, "data"=w1100:string[][], "NI_report out"=w1114:refnum<class "NI_report.lvclass">, "left edge output cluster"=w1097:cluster{"row":i32, "column":i32})  [unwired: 5 in, 1 out]
        n444 = Array Subset(array=w1100, index (col)=2 ("index")) -> (w1098:string[][])  [unwired: 3 in]
        n445 = local write "Sonde Data Array"(w1098) -> ()
        n446 = call "find last occupied cell.vi"("data"=w1098, "Active Sheet"=w1095, "Header Rows to remove"=3, "sub array start"=w1097, "error in (no error)"=w1115) -> ("row max value"=w1096:i32, 13:"start of last occupied row"=w1105:cluster{"row":i32, "column":i32}, 14:"start of last occupied row"=w1094:string, "error out"=w1088:errorcluster)  [unwired: 4 in, 3 out]
        n447 = local write "row max value"(w1096) -> ()
        n448 = local write "last occupied cell's name"(w1094) -> ()
      }
      frame "Init" {
        n449 = flat-sequence {
          tunnel: w1143 -> [w1173]
          tunnel: [w1164] -> w1141
          tunnel: [w1159] -> w1144
          frame #0 {
            n450 = call "create DAQ strings.vi"("error in (no error)"=w1173, "MCC USB-DAQ Setup"="MCC USB-DAQ Setup") -> ("error IO"=w1166:errorcluster, "Descriptions"=w1162:string[], "delimited string"=w1167:string, "Array"=w1163:string[], "Voltage Range"=w1172:dbl[])  [unwired: 5 in]
            "delimited string" <- w1167
            "Active Channel Array" <- w1163
            "Voltage Range" <- w1172
            "Descriptions" <- w1162
            n451 = call "Physical Channels to Number of channels.vi"("error in (no error)"=w1166, "Physical Channel in"=w1167) -> ("error out"=w1168:errorcluster, "Number of Channels"=w1170:i32)  [unwired: 7 in, 1 out]
            "Number of Channels" <- w1170
            n452 = call "Calculate Rate from Num Channels and Max Rate.vi"("error in (no error)"=w1168, "Channel Data Rate S/s"="Channel Data Rate S/s", "Number of Channels"=w1170) -> ("error out"=w1160:errorcluster, "Rate"=→"Rate":dbl)  [unwired: 7 in]
            n453 = for {
              tunnel: w1163 -> [w1180] mode=indexing
              tunnel: w1172 -> [w1179] mode=indexing
              tunnel: [w1176] -> w1159 mode=indexing
              shift-right: [w1177] -> w1165
              shift-left: w1160 -> [w1175]
              n454 = Negate(x=w1179) -> (-x=w1178:dbl)
              n455 = call-poly <vilib>:"ULx Create Virtual Channel.vi"("maximum value"=w1179, "minimum value"=w1178, "physical channels"=w1180, "error in"=w1175) -> ("task out"=w1176:refnum<k24>, "error out"=w1177:errorcluster)  [unwired: 10 in]
            }
            n456 = call "get 9V monitor voltage.vi"("error in (no error)"=w1165, "Descriptions"=w1162, "Array"=w1163, "Array 2"=w1159) -> ("error out"=w1164:errorcluster, "9V Voltage Monitor"=→"9V Voltage Monitor":dbl)  [unwired: 6 in]
            "DAQ Error" <- w1164
          }
        }
        n457 = flat-sequence {
          tunnel: w1141 -> [w1152]
          tunnel: [w1152] -> w1140
          frame #0 {
            w1153 = T18."Enabled" ("Disabled")
            n458 = property on="Write Data to Spreadsheet" class="Bool"("DisabledEnum"=w1153) -> (error out=w1156:errorcluster)  [unwired: 2 in, 1 out]
            n459 = property on="Record Continuous Samples" class="Bool"(error in=w1156, "DisabledEnum"=T18."Disabled and Grayed Out" ("Disabled")) -> (error out=w1155:errorcluster)  [unwired: 1 in, 1 out]
            n460 = property on="Record Single Sample" class="Bool"(error in=w1155, "DisabledEnum"=w1153) -> (error out=w1154:errorcluster)  [unwired: 1 in, 1 out]
            n461 = property on="Sample Not Collected" class="Bool"(error in=w1154, "DisabledEnum"=w1153) -> ()  [unwired: 1 in, 2 out]
            "Initialization Finished" <- TRUE
          }
        }
      }
      frame "Acq. DAQ data" {
        n462 = for {
          tunnel: w1184 -> [w1198] mode=indexing
          tunnel: w1183 -> [w1197]
          tunnel: [w1195] -> w1181 mode=indexing
          tunnel: [w1194] -> _ mode=indexing
          tunnel: [w1193] -> w1182 mode=indexing
          n463 = call-poly <vilib>:"ULx Read.vi"("task in"=w1198, "timeout"=10.0, "error in"=w1197) -> ("task out"=w1195:refnum<k24>, "data"=w1193:dbl, "error out"=w1194:errorcluster)  [unwired: 10 in]
        }
        "Raw Voltages" <- w1182
      }
      frame "Exit" {
        n464 = case shown="No Error" w1203 {
          tunnel: w1199 -> [w1239 _]
          tunnel: w1203 -> [w1238 w1250]
          tunnel: [w1237 w1250] -> w1201
          frame No Error {
            n465 = for {
              shift-right: [w1241] -> w1237
              shift-left: w1238 -> [w1242]
              tunnel: w1239 -> [w1240] mode=indexing
              n466 = while {
                shift-right: [w1249] -> w1244
                shift-left: w1242 -> [w1247]
                shift-right: [w1248] -> w1243
                shift-left: w1240 -> [w1246]
                stop <- w1245 stop-if-true
                n467 = call <vilib>:"ULx Is Task Done.vi"("task in"=w1246, "error in"=w1247) -> ("task out"=w1248:refnum<k24>, "task done?"=w1245:bool, "error out"=w1249:errorcluster)  [unwired: 11 in]
              }
              n468 = call <vilib>:"ULx Clear Task.vi"("task in"=w1243, "error in"=w1244) -> ("error out"=w1241:errorcluster)  [unwired: 13 in]
            }
          }
          frame Error {
          }
        }
        n469 = local read "report file path"() -> (w1216:path)
        n470 = flat-sequence {
          tunnel: [w1256] -> w1210
          tunnel: [w1255] -> w1213
          tunnel: w1212 -> [w1253]
          tunnel: w1211 -> [w1252]
          tunnel: w1216 -> [w1251]
          frame #0 {
            n471 = call-dynamic "Save Report to File.vi"("report in"=w1252, "report file path"=w1251, "prompt to replace? (F)"=FALSE, "error in (no error)"=w1253) -> ("report out"=w1256:refnum<class "NI_report.lvclass">, "error out"=w1255:errorcluster)  [unwired: 10 in]
          }
        }
        n472 = call <userlib>:"Wait (ms)__ogtk.vi"("error in (no error)"=w1213, "milliseconds to wait"=u32 5) -> ("error out"=w1214:errorcluster)  [unwired: 8 in, 1 out]
        n473 = flat-sequence {
          tunnel: w1214 -> [w1225]
          tunnel: w1210 -> [w1223]
          tunnel: [w1221] -> w1204
          frame #0 {
            (unwired) FALSE ("Write Ini")
            n474 = call-dynamic "Dispose Report.vi"("report in"=w1223, "save changes? (F)"=FALSE, "error in (no error)"=w1225) -> ("error out"=w1220:errorcluster)  [unwired: 12 in]
            n475 = case shown="False" "Save Configuration File?" {
              tunnel: [errorcluster {"status"=FALSE, "code"=0, "source"=""} ("error IO") w1234] -> w1222
              frame False {
              }
              frame True {
                n476 = local read "Config File Path"() -> (w1233:path)
                n477 = call <vilib>:"Open Config Data.vi"("create file if necessary (T)"=TRUE ("Read Ini"), "configuration file path"=w1233) -> ("error out"=w1231:errorcluster, "refnum"=w1228:T17)  [unwired: 7 in, 1 out]
                n478 = control-ref of="This VI"() -> (w1227:refnum<vi>)
                n479 = call <userlib>:"Write Panel to INI__ogtk.vi"("error in (no error)"=w1231, "VI ref"=w1227, "refnum"=w1228) -> ("error out"=w1230:errorcluster, "refnum out"=w1229:T17)  [unwired: 7 in]
                n480 = call <vilib>:"Clear Errors.vi"("error in (no error)"=w1230) -> ("error out"=w1236:errorcluster)  [unwired: 5 in, 1 out]
                n481 = call <vilib>:"Close Config Data.vi"("error in (no error)"=w1236, "refnum"=w1229) -> ("error out"=w1235:errorcluster)  [unwired: 8 in, 1 out]
                n482 = Merge Errors(w1235, w1230) -> (w1234:errorcluster)
              }
            }
            n483 = Merge Errors(w1222, w1220) -> (w1221:errorcluster)
          }
        }
        n484 = flat-sequence {
          tunnel: [TRUE ("aborted?")] -> w1202
          tunnel: [w1217] -> w1200
          tunnel: w1201 -> [w1217]
          frame #0 {
          }
        }
      }
    }
    "Stop 2" <- w320
    n485 = call "kpro 2016.vi"() -> ()  [unwired: 11 in, 5 out]
    "consumer loop" <- w348
  }
  "Feet of\nStainless to be\nUsed (Count)" <- w2
  "Feet of Stainless 2" <- w1
  n486 = Merge Errors(w29, w28) -> (→"error out":errorcluster)
